vi "mainCryo With New Driver V1 and Cri Modified by Patiwet.vi"() -> ()   [LabVIEW 2012]
uses:
  SubVI/ProSCI Global.vi
  HTB/priorlibfilterout.vi
  <vilib>/Utility/config.llb/Write Key (I32).vi
  <vilib>/Utility/config.llb/Write Key (U32).vi
  <vilib>/Instr/_visa.llb/VISA Configure Serial Port (Instr).vi
  SubVI/ProSCI ConfigGlobal.vi
  <vilib>/Utility/config.llb/Read Key (U32).vi
  <vilib>/Utility/config.llb/Read Key (I32).vi
  <vilib>/Utility/config.llb/Read Key (Double).vi
  <vilib>/Utility/config.llb/Write Key (String).vi
  <vilib>/Utility/config.llb/Read Key (String).vi
  HTB/priorlibscanout.vi
  SubVI/ProSCI DebugGlobal.vi
  <vilib>/Utility/config.llb/NI_LVConfig.lvlib
panel:
  in  "stop":bool
  in  "port 2":i32=3
  in  "Case Constant\n(See Context Help) 3":bool
  in  "Case Constant\n(See Context Help) 2":bool
  in  "Case Constant\n(See Context Help)":bool=TRUE
  out "ExpTime":string
  out "ExpDate":string
  out "Event":i32(listbox)
  out "BotEdgePos":i32
  out "TopEdgePos":i32
  out "RtEdgePos":i32
  out "LtEdgePos":i32
  out "EdgeMarker":u8
  out "RobotIndexed":bool
  out "TotROI":i32
  out "TempXYArray":i32[](array[numeric])
  out "TileXYCoordinates":i32[][](array[numeric])
  out "Mag":u8
  out "Obj":u8
  out "CameraCounter":u32
  out "Br VISA Ref":refnum<visa-resource-name>="COM2"
  out "InGoHomeState":u32
  out "GoingHome":bool=TRUE
  out "CutCompXition":bool
  out "BaseDir":string
  in  "Tab Control":T1(tab)=enum."Imaging"
  in  "SampleThk":u32 max=70 step=1
  out "SecNumInFile":u32
  out "NotifyAbout":T2(ring)
  in  "Notify":bool
  out "UpdateMetadata":bool
  in  "PI":string
  in  "User":string
  out "ImageNow":bool
  out "TotalSessionCuts":u32
  out "SaveMetadata":bool
  in  "OpNotes":string
  in  "OpSliceThk":u16 max=50 step=1
  in  "OpSpecimen":string
  out "Present Cuts":u32
  in  "Total Cuts":u32
  out "Sequence Cut":bool
  in  "Image":bool
  out "IO Cut Comp":bool
  in  "FluoExpArray":dbl[](array[numeric])
  out "CutsCompletedLast":u32
  in  "ImageType":u16(ring) items=["Brightfield Only", "Fluorescence Only", "Brightfield & Fluorescence"]
  in  "ImageInterval":i32 min=0 max=25
  in  "IntervalMode":u16(ring) items=["Brightfield", "Fluorescence"]
  out "FlExpMem":dbl format="%#.3f"
  out "BrExpMem":dbl format="%#.3f"
  in  "FileNumStart":i32=1 min=0 max=10000
  in  "ImageSkipNum":i32 min=0 max=50
  in  "Capture Single Image":bool
  in  "ImageRepeatNum":u32=1 min=1
  out "FullFileName":string
  in  "SetFile Button":bool
  in  "FileNumbering":enum32{"Continuous", "With Section No."}(radio)=enum."With Section No."
  out "AutoXOffset":i32
  out "OffsetSlice":u32
  in  "OffsetPx":u32=1 min=1 step=1
  in  "Auto Offset":bool
  out "Pixel Size":dbl
  out "OffsetPresent":bool
  in  "ClearGlobalOffset":bool
  in  "StoreGlobalOffset":bool
  in  "Image ROI":bool
  in  "RobotStop":bool
  in  "BotEdge":bool
  in  "RightEdge":bool
  in  "LeftEdge":bool
  in  "TopEdge":bool
  out "Robot State":T3(ring)
  in  "RobotJog":bool
  in  "Magnification":string(combo)
  in  "Objective":string(combo)
  in  "Tile ROI":bool
  in  "MoveTo ROI":bool
  in  "Delete ROI":bool
  in  "Rename ROI":bool
  in  "Add ROI":bool
  in  "ROIName":string
  in  "ROI List":i32(listbox)
  in  "RobotFocus":bool
  in  "RobotImage":bool
  in  "RobotPark":bool
  in  "RobotIndex":bool
  out "RobotOnline":bool
  in  "RobotDisConnect":bool
  in  "RobotConnect":bool
  out "FlConnection":bool
  in  "Lamp Delay":dbl=2.0 min=0.5 max=5.0 step=0.1 format="%#.1f"
  in  "Shutter On":bool
  in  "BrDisonnectButton":bool
  in  "BrConnectButton":bool
  in  "FlDisonnectButton":bool
  in  "FlConnectButton":bool
  in  "FlIntensityLevel":u8(ring) items=["0%"=1, "11%"=2, "22%"=3, "33%"=4, "44%"=5, "55%"=6, "66%"=7, "77%"=8, "88%"=9, "100%"=10]
  out "BrLampStatus":T4(ring)
  out "BrConnection":bool
  out "BrFWVer":string
  in  "Lamp On":bool
  in  "Intensity":u8=100 max=100 step=10
  in  "Robot VISA Ref":refnum<visa-resource-name>
  out "Debug":string
  in  "Image Delay (sec)":dbl=2.0 format="%#_1g"
  in  "RobotIdx":bool
  in  "EProfile":bool
  in  "MinOverlap":bool
  out "LubBase":i32
  out "KnifeBase":i32
  in  "SaveFocusData":bool
  in  "Overlap":u8=15 min=5 max=90 step=1
  out "Camera Prog. OK":bool
  in  "Sys Reset":bool
  in  "Time Out (sec)":dbl=80.0 format="%#_1f"
  out "IO Fwd Stroke":bool
  in  "ResetLub":bool
  in  "ResetKnife":bool
  out "KnifeTime":i32
  out "LubTime":i32
  out "LubSetTime":u32=120 format="%#_3f"
  out "KnifeSetTime":u32=165 format="%#_3f"
  out "Lubricate":bool
  out "Change Knife":bool
  out "MBT Function: ErrorOut":errorcluster {"code" format="%.0x"}
  in  "AbortSeq":bool
  out "StXition":bool
  out "Current State":T5(ring)
  out "Imaging Done":bool
  in  "Single":bool
  in  "Sequence":bool
  in  "PauseReset":bool
  in  "Home":bool
  out "InFwdState":u32
  out "InDelayState":u32
  in  "Go Home Output":bool
  in  "Stop Cut Output":bool
  in  "Start Cut Output":bool
  out "Go Home":bool
  out "Stop Cut":bool
  out "Start Cut":bool
  out "IO EStop?":bool
  out "IO Comp Mode?":bool
  # "Op Exp Time - Remove Later"
  # "Emergency Stop?"
  # "In Computer Mode?"
  # "EVENT LOG"
  # "CONTROL"
  # "SETUP"
  # "STATUS"
  # "Experiment Details"
  # "Section Thickness"
  # "microns"
  # "Sample Thickness"
  # "mm"
  # "Notes"
  # "Cut Complete Signal"
  # "Sequence Cut"
  # "Total Cuts in Sequence"
  # "Image File #"
  # "Total Cuts This Session"
  # "Specimen"
  # "Cuts Completed"
  # "Only Sectioning"
  # "Section and Image"
  # "Skip Imaging every"
  # "Section(s)"
  # "Start File Numbering at"
  # "Base Image File Name"
  # "Images Per Section"
  # "Memorized BF Exposure Time"
  # "Memorized FL Exposure Time"
  # "msec"
  # "msec"
  # "Additional Fluo Exposures\n(Green Channel Only)"
  # "Select Image Type"
  # "Take"
  # "Image at Interval of"
  # "File Numbering"
  # "Robot Control"
  # "Scope Settings"
  # "Magnification"
  # "Objective"
  # "um"
  # "ROI/Tile Settings"
  # "New ROI"
  # "Selected ROI"
  # "FOV Offset"
  # "Manual"
  # "@"
  # "pixels"
  # "sections"
  # "Brightfield"
  # "Connection"
  # "Firmware Version"
  # "Lamp Unit Status"
  # "sec"
  # "Fluorescence"
  # "Connection"
  # "Firmware Version"
  # "Lamp Hours"
  # "Intensity Level"
  # "Mechanical"
  # "Miscellany"
  # "Change Knife every"
  # "IP: 169.254.0.101"
  # "Modbus TCP/IP"
  # "sections"
  # "Total Knife Run"
  # "sections"
  # "Change Knife?"
  # "Lubricate Machine every"
  # "sections"
  # "Total Lub Run Time"
  # "sec"
  # "Wait"
  # "sections"
  # "before Imaging"
  # "Lub Machine?"
  # "Tiling/ROI/Robot"
  # "Cut Complete Timeout"
  # "New Focus Data"
  # "seconds"
  # "Min Tile Overlap"
  # "%"
  # "Keep Overlap at Minimum"
  # "Robot Profile"
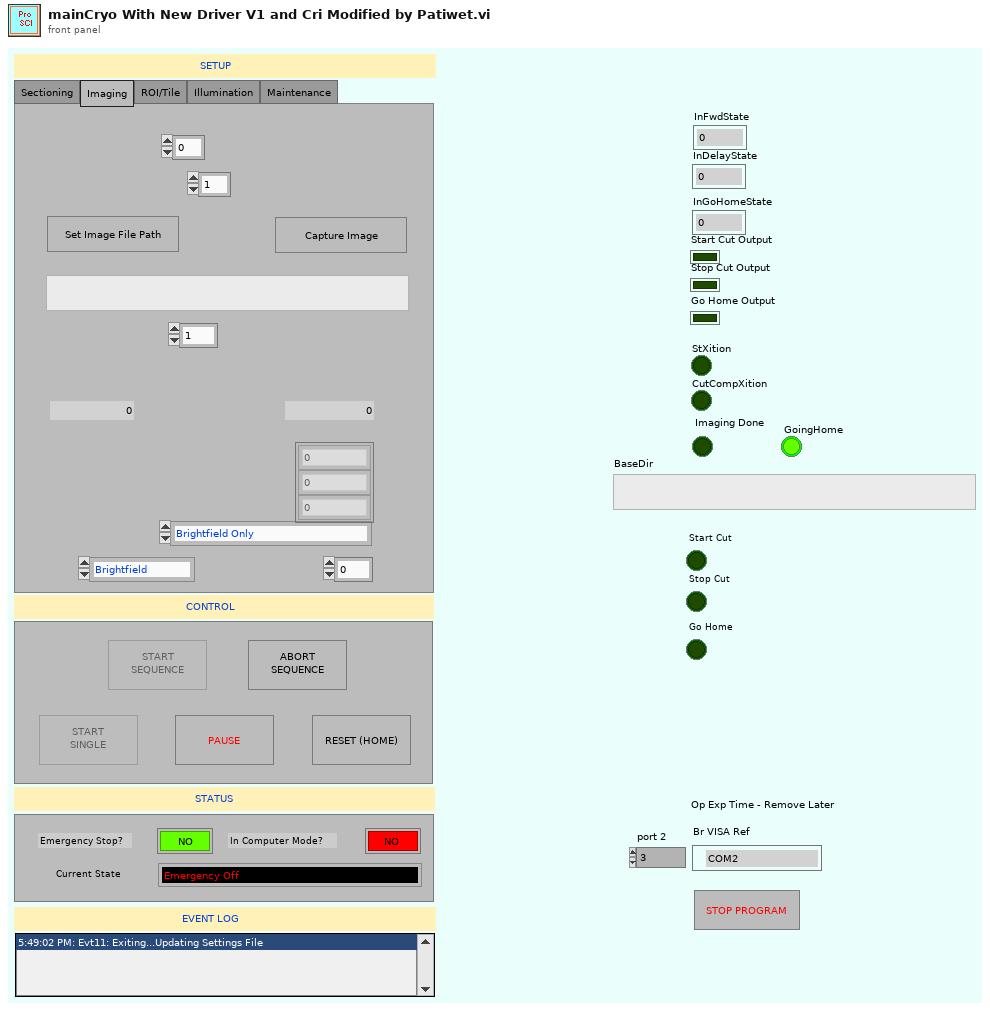
[diagram p1: front panel]
types:
  T1 = enum32{"Sectioning", "Imaging", "ROI/Tile", "Illumination", "Maintenance"}
  T2 = enum16{"Nothing", "In Progress", "Aborted", "Completed", "Sec TO"}
  T3 = enum16{"Idle", "Jog", "Indexing", "Parking", "Moving to Image", "Focusing", "Moving to ROI", "Not Indexed", "Offline"}
  T4 = enum16{"Undefined", "Connection Lost", "Not in Remote Mode", "Replace Bulb", "Lamp Unit OK"}
  T5 = enum16{"Emergency Off", "Manual", "Idle", "Spare 1", "Forward", "Pause", "Go Home", "Spare 2", "Cut Complete", "Imaging", "Spare 3", "Calculate Cuts", "Spare 4", "Time Out", "Delay Before Imaging"}
  T6 = enum16{"open", "open or create", "create or replace", "create", "open (read only)"}
  T7 = typedef "LVRectTypeDef.ctl" = cluster{"Left":i16, "Top":i16, "Right":i16, "Bottom":i16}
  T8 = typedef "NI_LVConfig.lvlib/Config Data RefNum.ctl" = refnum<k1>
  T9 = enum32{"existing file", "new file", "new or existing file", "existing dir", "new dir", "new or existing dir", "existing file (use LLBs)", "new file (use LLBs)", "new or existing file (use LLBs)", "new or existing file or directory (use LLBs)"}
  T10 = cluster{"PI":string, "User":string, "OpSpecimen":string, "OpSliceThk":u16, "OpNotes":string, "Image":bool}
  T11 = cluster{"ImageSkipNum":i32, "FileNumStart":i32, "FileNumbering":enum32{"Continuous", "With Section No."}, "FullFileName":string, "BaseDir":string, "ImageRepeatNum":u32, "BrExpMem":dbl, "FlExpMem":dbl, "ImageType":u16, "IntervalMode":u16, "ImageInterval":i32}
  T12 = cluster{"Obj":u8, "Mag":u8, "ItemNames":string[][], "TileXYCoordinates":i32[][], "TotROI":i32}
  T13 = cluster{"Time Out (sec)":dbl, "Overlap":u8, "MinOverlap":bool, "EProfile":bool, "Image Delay (sec)":dbl}
  T14 = enum16{"Undefined", "Focus", "XMin", "YMax", "XY", "Exposure"}
  T15 = enum16{"Idle", "Jog", "Indexing", "Parking", "Moving to Image", "Focusing", "Moving to ROI"}
  T16 = enum16{"Idle", "Jog", "Indexing", "Parking", "Moving to Image", "Focusing", "Moving to ROI", "Not Indexed"}
  T17 = enum16{"Add", "Delete", "Rename", "Update Tiles"}
  T18 = enum16{"Undefined", "Focus", "XMin", "YMax", "XY"}
  T19 = enum16{"Nothing", "In Progress", "Aborted", "Completed"}
  T20 = cluster{"TileCoordinates":i32[][], "XTiles":u16, "YTiles":u16, "TileSuffix":string[], "XOverlap":dbl, "YOverlap":dbl}
  T21 = cluster{"User":string, "PI":string, "OpSpecimen":string, "OpSliceThk":u16, "OpNotes":string, string, string}
  T22 = enum32{"invalid app kind", "Development System", "Run Time System", "Student Edition", "Embedded LabVIEW", "Evaluation", "Custom"}
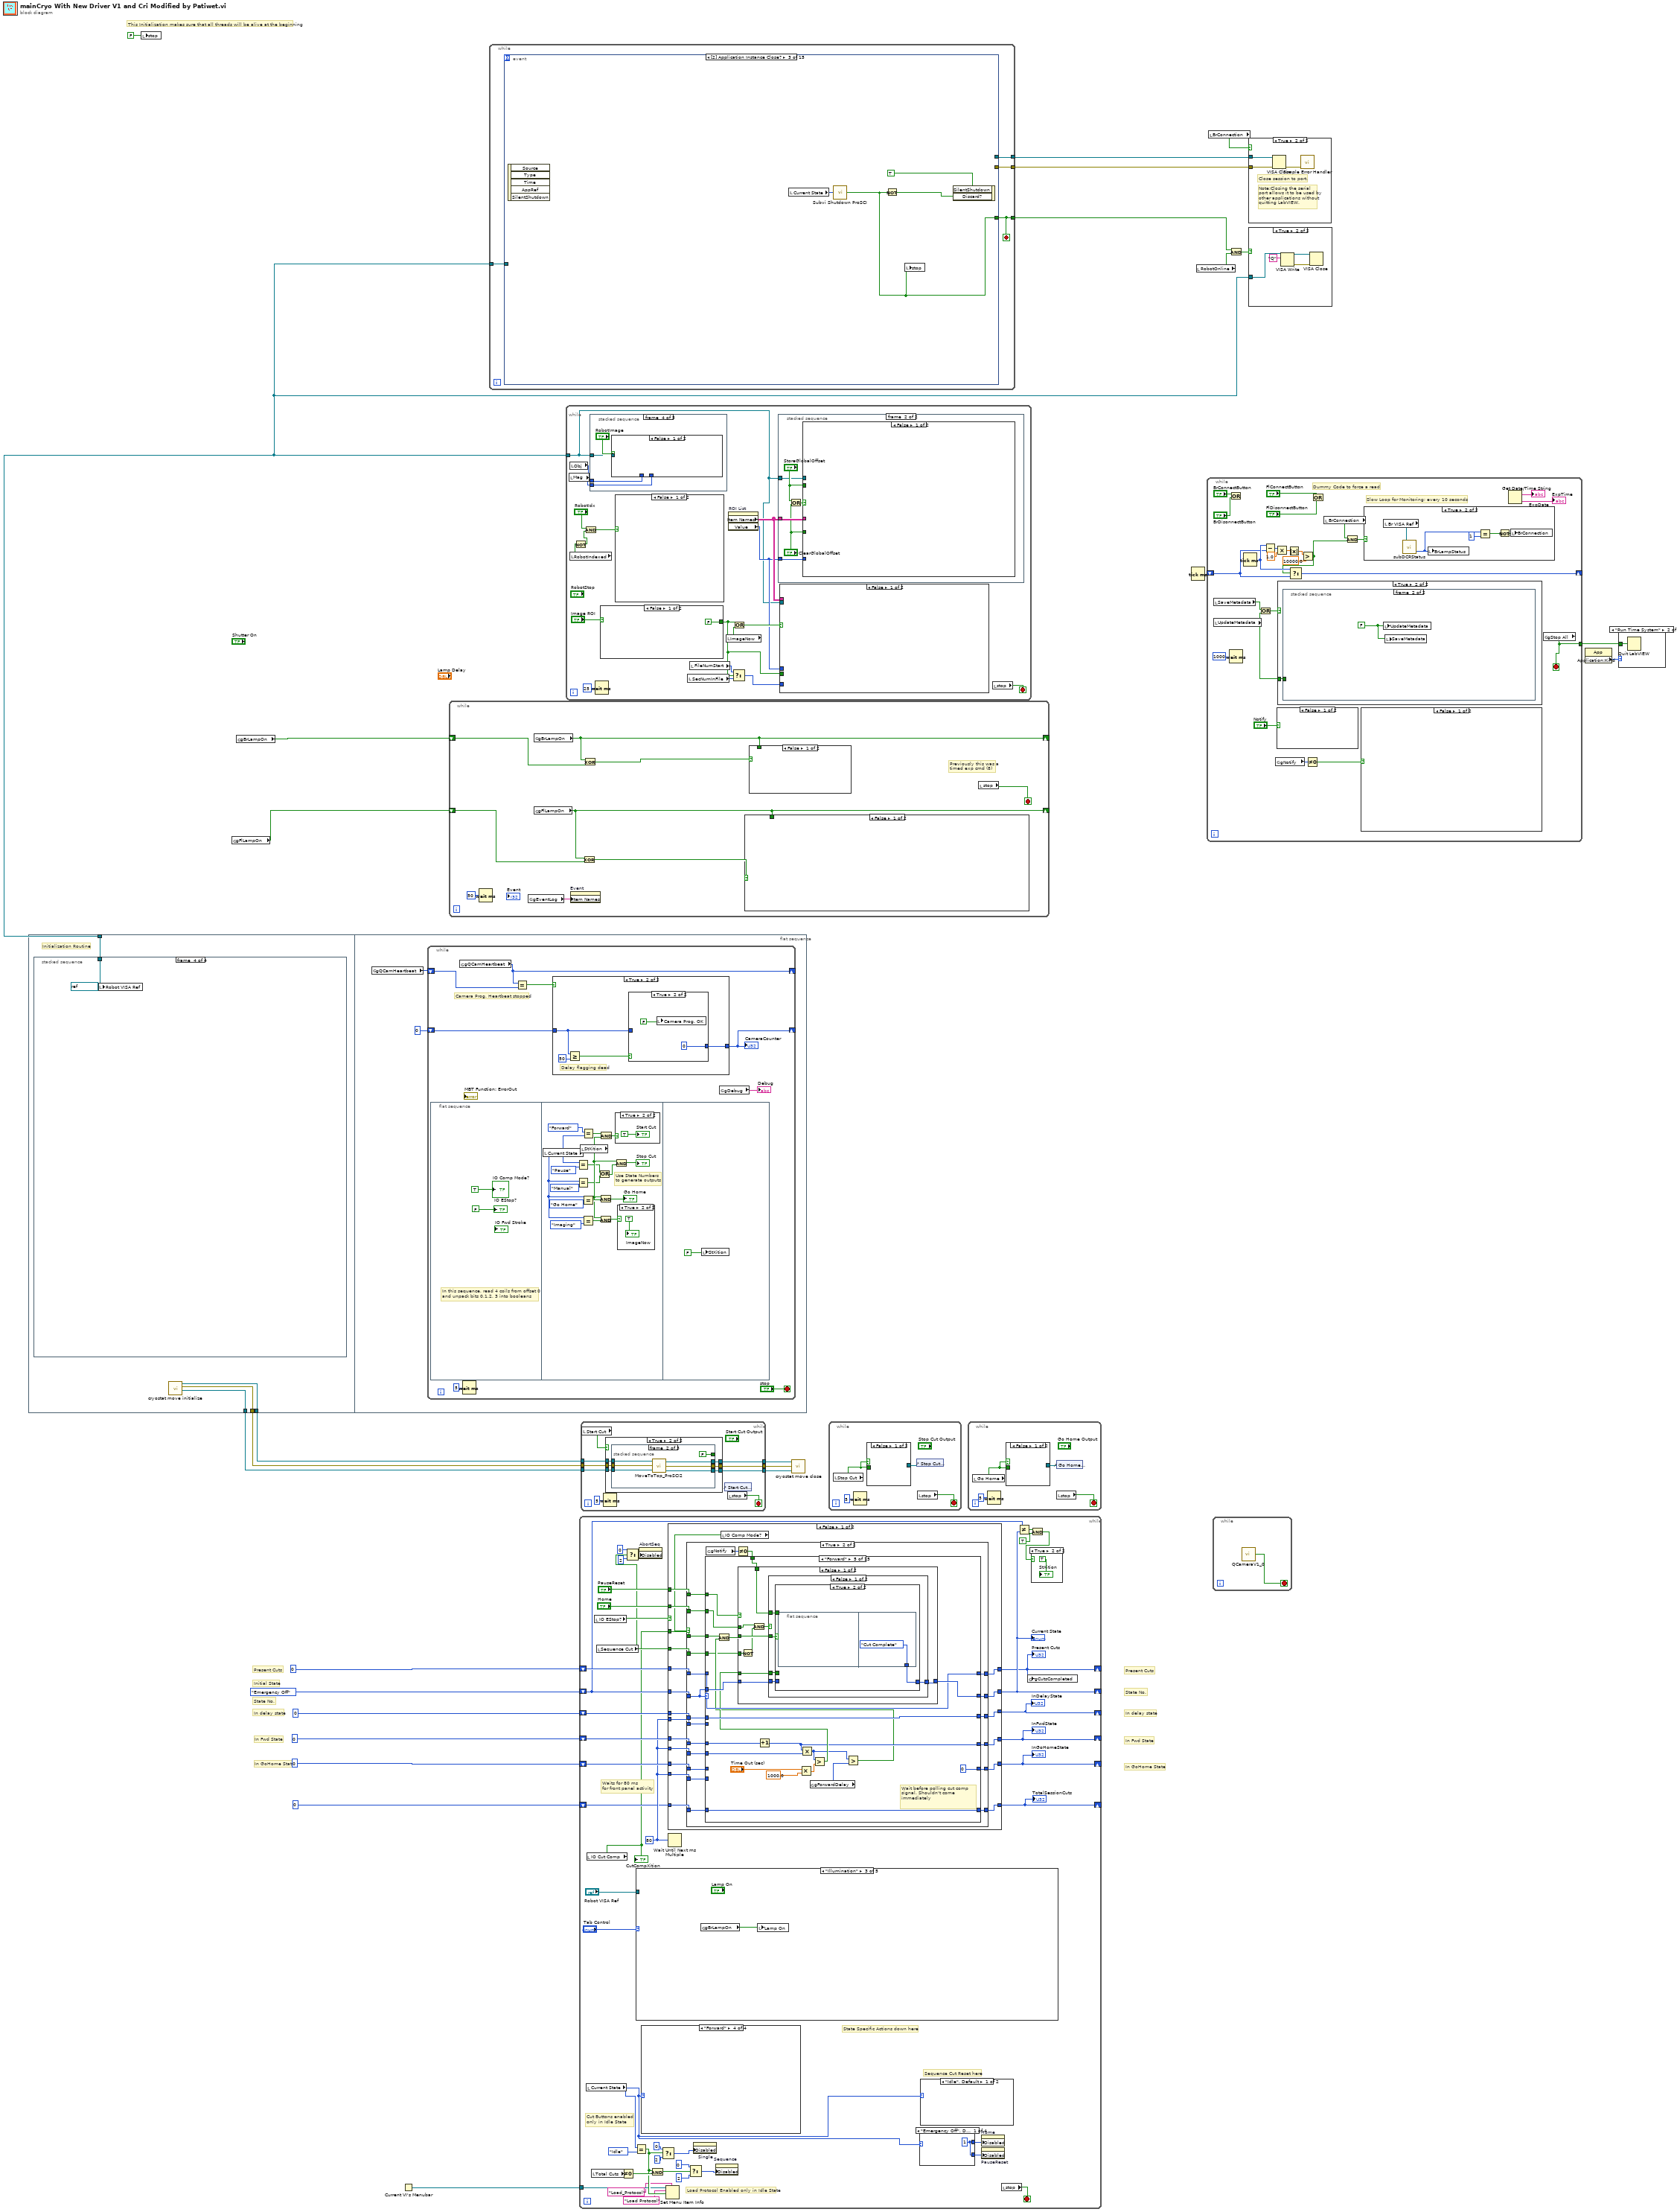
[diagram p0: block diagram]
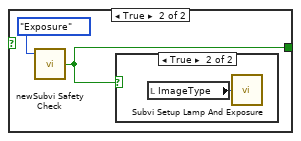
[diagram p5: hidden frame]
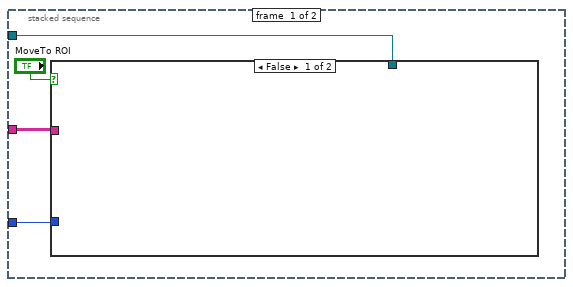
[diagram p7: hidden frame]
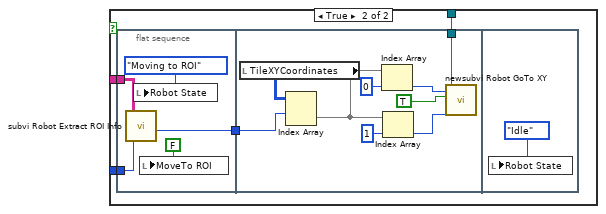
[diagram p8: hidden frame]
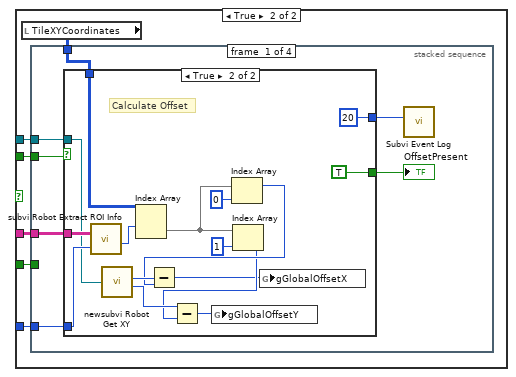
[diagram p9: hidden frame]
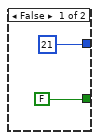
[diagram p10: hidden frame]
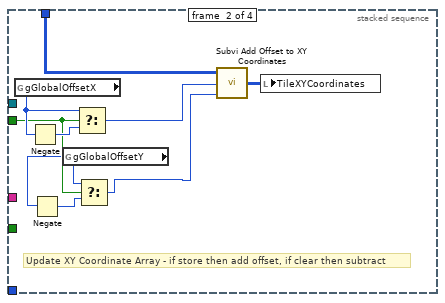
[diagram p11: hidden frame]
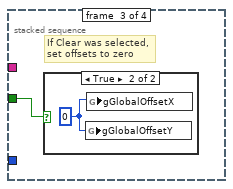
[diagram p12: hidden frame]
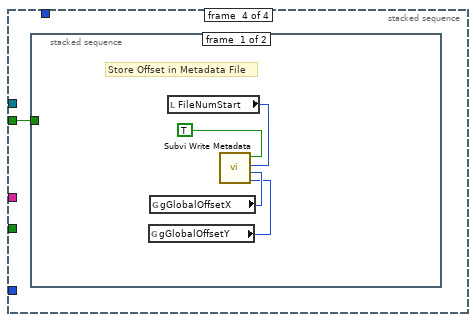
[diagram p14: hidden frame]
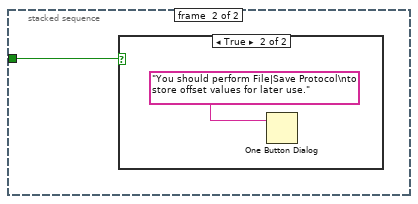
[diagram p15: hidden frame]
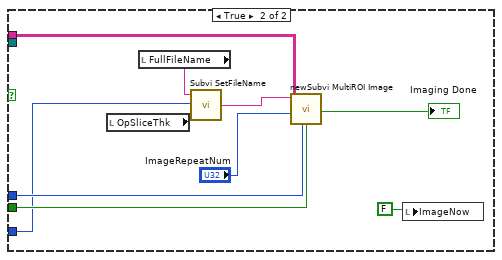
[diagram p17: hidden frame]
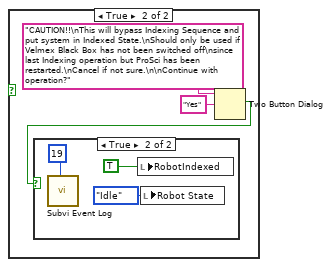
[diagram p18: hidden frame]
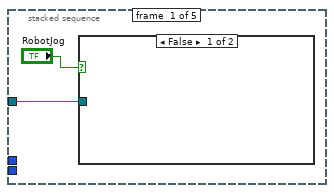
[diagram p20: hidden frame]
diagram:
  # "This Initialization makes sure that all threads will be alive at the beginning"
  # "In GoHome State"
  # "In GoHome State"
  # "In Fwd State"
  # "In Fwd State"
  # "Present Cuts"
  # "Present Cuts"
  # "State No."
  # "In delay state"
  # "In delay state"
  # "State No."
  # "Initial State"
  n1 = flat-sequence {
    tunnel: [w30] -> w9
    tunnel: [w29] -> w6
    tunnel: [w28] -> w5
    tunnel: [w27] -> w4
    frame #0 {
      # "Initialization Routine"
      n2 = stacked-sequence {
        tunnel: [_ _ _ w107] -> w30
        frame #0 {
          w43 = i16 0
          # "Open Logfile"
          # "Window Size, Title"
          n3 = property class="VI"() -> ("Front Panel Window:Window Bounds"=w39:T7)  [unwired: 2 in, 2 out]
          n4 = Current VI's Path() -> (path=w34:path)
          n5 = Strip Path(path=w34) -> (stripped path=w32:path)  [unwired: 1 out]
          n6 = Strip Path(path=w32) -> (stripped path=w31:path)  [unwired: 1 out]
          n7 = Unbundle(w39) -> ("Right"=w42:i16, "Bottom"=w41:i16)  [unwired: 2 out]
          n8 = Bundle(w43, w43, "Right"=w42, "Bottom"=w41) -> (w40:cluster{i16, i16, "Right":i16, "Bottom":i16})  [unwired: 1 out]
          n9 = Concatenate Strings("Pro-SCI" ("string"), " - Untitled" ("string")) -> (w46:string)
          n10 = property class="VI"("Front Panel Window:Window Bounds"=w40, "Front Panel Window:Title"=w46) -> ()  [unwired: 2 in, 2 out]
          n11 = call "Subvi SetLogFileName.vi"("LogFileMax"=u8 10 ("y"), "BaseAppPath"=w31, "LogFileBaseName"="ProSCILog") -> ("LogFilePath"=w33:path)
          n12 = call <vilib>:"Open_Create_Replace File.vi"("function (open:0)"=T6."open or create", "file path"=w33) -> ("refnum"=w37:refnum<file>)  [unwired: 4 in, 5 out]
          n13 = global write "ProSCI Global.vi" "gLogFileRef"(w37) -> ()
        }
        frame #1 {
          w50 = "D:\\Default" ("string")
          w55 = string[] [] ("Item Names")
          w48 = u8 0 ("gAppsStopped")
          w60 = FALSE
          w62 = u8 0 ("Disabled")
          n14 = local write "TileXYCoordinates"(i32[][] [] ("TileXYCoordinates")) -> ()
          n15 = local write "TempXYArray"(i32[] [] ("TempXYArray")) -> ()
          n16 = global write "ProSCI Global.vi" "gStop All"(w60) -> ()
          n17 = global write "ProSCI Global.vi" "gCutSequenceOn"(w60) -> ()
          n18 = local write "BaseDir"(w50) -> ()
          n19 = property on="ROI List" class="MCListbox (strict)"("Item Names"=string[][] []) -> ()  [unwired: 2 in, 2 out]
          n20 = global write "ProSCI Global.vi" "gBaseDir"(w50) -> ()
          n21 = Concatenate Strings(w50, "\\CryoDefault" ("string")) -> (w51:string)
          n22 = local write "Tab Control"(T1."Sectioning" ("Tab Control")) -> ()
          n23 = local write "FullFileName"(w51) -> ()
          n24 = global write "ProSCI Global.vi" "gBaseFile"(w51) -> ()
          n25 = property on="TopEdge" class="Bool"("Visible"=w60) -> ()  [unwired: 2 in, 2 out]
          n26 = property on="BotEdge" class="Bool"("Visible"=w60) -> ()  [unwired: 2 in, 2 out]
          n27 = property on="Magnification" class="CmbBox"("Value"="0" ("Magnification")) -> ()  [unwired: 2 in, 2 out]
          n28 = global write "ProSCI Global.vi" "gEventLog"(w55) -> ()
          n29 = property on="Event" class="LstBox (strict)"("Item Names"=w55) -> ()  [unwired: 2 in, 2 out]
          n30 = property on="RightEdge" class="Bool"("Visible"=w60) -> ()  [unwired: 2 in, 2 out]
          n31 = property on="LeftEdge" class="Bool"("Visible"=w60) -> ()  [unwired: 2 in, 2 out]
          n32 = property on="Objective" class="CmbBox"("Value"="0" ("Objective")) -> ()  [unwired: 2 in, 2 out]
          n33 = To Double Precision Float(number=w48) -> (double precision float=w49:dbl)
          n34 = local write "FlIntensityLevel"(10) -> ()
          n35 = property on="FlConnectButton" class="Bool (strict)"("Disabled"=w62) -> ()  [unwired: 2 in, 2 out]
          n36 = property on="BrDisonnectButton" class="Bool (strict)"("Disabled"=w62) -> ()  [unwired: 2 in, 2 out]
          n37 = property on="BrConnectButton" class="Bool (strict)"("Disabled"=w62) -> ()  [unwired: 2 in, 2 out]
          n38 = property on="FlDisonnectButton" class="Bool (strict)"("Disabled"=w62) -> ()  [unwired: 2 in, 2 out]
          n39 = global write "ProSCI Global.vi" "gExpTimeSendToCamera"(w49) -> ()
          n40 = local write "EdgeMarker"(w48) -> ()
          n41 = global write "ProSCI Global.vi" "gAppsStopped"(w48) -> ()
          n42 = local write "TotROI"(w48) -> ()
          "Robot State" <- T3."Offline" ("Robot State")
        }
        frame #2 {
          w75 = "Robot" ("section")
          w87 = "Mechanical" ("section")
          # "This number should always be negative"
          # "Row = Magnification\nCol = Objective"
          # "in microns"
          # "90x"
          # "7x"
          # "1.0X"
          # "0.3X"
          # "Later replace this part by reading the same settings from Settings file"
          # "Read from Settings File"
          n43 = String To Path(string="C:\\Program Files\\ProSCI\\ProSciSettings.ini") -> (path=w102:path)
          n44 = call <vilib>:"Open Config Data (compatibility).vi"("create file if necessary (T)"=FALSE ("create file if necessary? (T)"), "configuration file path"=w102) -> ("error out"=w98:errorcluster, "refnum"=w100:T8)  [unwired: 7 in, 1 out]
          n45 = call-poly <vilib>:"Read Key.vi"("section"=w87, "error in (no error)"=w98, "default value"=u32 0, "key"="ChangeKnife", "refnum"=w100) -> ("error out"=w91:errorcluster, "value"=→"KnifeSetTime":u32, "refnum out"=w92:T8)  [unwired: 4 out]
          n46 = call-poly <vilib>:"Read Key.vi"("section"=w87, "error in (no error)"=w91, "default value"=0, "key"="KnifeRun", "refnum"=w92) -> ("error out"=w89:errorcluster, "value"=w79:i32, "refnum out"=w90:T8)  [unwired: 4 out]
          "KnifeBase" <- w79
          n47 = global write "ProSCI ConfigGlobal.vi" "gCfgPixelSize"(dbl[][] [[52.0, 15.6], [41.2, 11.0], [29.3, 8.8], [24.0, 7.2], [18.0, 5.4], [15.4, 4.6], [11.7, 3.5], [9.6, 2.9], [7.1, 2.1], [5.3, 1.6], [4.0, 1.2]] ("array")) -> ()
          n48 = local write "KnifeTime"(w79) -> ()
          n49 = call-poly <vilib>:"Read Key.vi"("section"=w87, "error in (no error)"=w89, "default value"=u32 0, "key"="LubMachine", "refnum"=w90) -> ("error out"=w83:errorcluster, "value"=→"LubSetTime":u32, "refnum out"=w86:T8)  [unwired: 4 out]
          n50 = call-poly <vilib>:"Read Key.vi"("section"=w87, "error in (no error)"=w83, "default value"=0, "key"="LubRun", "refnum"=w86) -> ("error out"=w76:errorcluster, "value"=w80:i32, "refnum out"=w77:T8)  [unwired: 4 out]
          "LubBase" <- w80
          n51 = call-poly <vilib>:"Read Key.vi"("section"=w75, "error in (no error)"=w76, "default value"=6.35, "key"="MicronPerStep" ("section"), "refnum"=w77) -> ("error out"=w73:errorcluster, "value"=w70:dbl, "refnum out"=w74:T8)  [unwired: 4 out]
          n52 = global write "ProSCI ConfigGlobal.vi" "gCfgMicronPerStep"(w70) -> ()
          n53 = call-poly <vilib>:"Read Key.vi"("section"=w75, "error in (no error)"=w73, "default value"=-0.267949, "key"="MicronPerMicronThickness" ("section"), "refnum"=w74) -> ("error out"=w66:errorcluster, "value"=w64:dbl, "refnum out"=w67:T8)  [unwired: 4 out]
          n54 = Greater Or Equal To 0?(x=w64) -> (x >= 0?=w65:bool)
          n55 = call <vilib>:"Close Config Data.vi"("error in (no error)"=w66, "write file if changed (T)"=FALSE ("write configuration file? (T)"), "refnum"=w67) -> ()  [unwired: 9 out]
          n56 = case shown="True" w65 {
            tunnel: w64 -> [w104 w106]
            tunnel: [w104 w105] -> w63
            frame False {
            }
            frame True {
              n57 = Negate(x=w106) -> (-x=w105:dbl)
            }
          }
          n58 = global write "ProSCI ConfigGlobal.vi" "gCfgMicronPerMicronThickness"(w63) -> ()
          n59 = local write "LubTime"(w80) -> ()
        }
        frame #3 {
          w107 = refnum<visa-resource-name> "COM8" ("Robot VISA Ref")
          n60 = local write "Robot VISA Ref"(w107) -> ()
        }
      }
      n61 = call "cryostat move initialize.vi"() -> ("VISA resource name out"=w27:refnum<visa-resource-name>, "error out 2"=w28:errorcluster, "task out"=w29:refnum<k21>)  [unwired: 8 in, 1 out]
    }
    frame #1 {
      n62 = global read "ProSCI Global.vi" "gQCamHeartbeat"() -> (w109:u32)
      n63 = while {
        shift-right: [w111] -> _
        shift-left: w109 -> [w115]
        shift-right: [w114] -> _
        shift-left: 0 -> [w113]
        stop <- "stop" stop-if-true
        # "Camera Prog. Heartbeat stopped"
        n64 = flat-sequence {
          frame #0 {
            # "In this sequence, read 4 coils from offset 0\nand unpack bits 0,1,2, 3 into booleans"
            "IO Comp Mode?" <- TRUE ("UseTCP")
            "IO EStop?" <- FALSE ("UseTCP")
          }
          frame #1 {
            # "Use State Numbers\nto generate outputs"
            n65 = local read "Current State"() -> (w135:T5)
            n66 = Equal?(x=w135, y=T5."Pause") -> (x = y?=w133:bool)
            n67 = Equal?(x=w135, y=T5."Manual") -> (x = y?=w132:bool)
            n68 = local read "StXition"() -> (w137:bool)
            n69 = Equal?(x=w135, y=T5."Go Home") -> (x = y?=w142:bool)
            n70 = Equal?(x=w135, y=T5."Imaging") -> (x = y?=w138:bool)
            n71 = Equal?(x=T5."Forward", y=w135) -> (x = y?=w145:bool)
            n72 = Or(x=w133, y=w132) -> (x .or. y?=w134:bool)
            n73 = And(x=w137, y=w142) -> (x .and. y?=→"Go Home":bool)
            n74 = And(x=w137, y=w138) -> (x .and. y?=w131:bool)
            n75 = And(x=w145, y=w137) -> (x .and. y?=w130:bool)
            n76 = And(x=w137, y=w134) -> (x .and. y?=→"Stop Cut":bool)
            n77 = case shown="True" w130 {
              frame False {
              }
              frame True {
                "Start Cut" <- TRUE
              }
            }
            n78 = case shown="True" w131 {
              frame False {
              }
              frame True {
                "ImageNow" <- TRUE
              }
            }
          }
          frame #2 {
            n79 = local write "StXition"(FALSE) -> ()
          }
        }
        n80 = global read "ProSCI Global.vi" "gQCamHeartbeat"() -> (w111:u32)
        n81 = Wait (ms)(milliseconds to wait=u32 5) -> ()  [unwired: 1 out]
        n82 = Equal?(x=w111, y=w115) -> (x = y?=w112:bool)
        n83 = case shown="True" w112 {
          tunnel: [0 w121] -> w114
          tunnel: w113 -> [_ w120]
          frame False {
            "Camera Prog. OK" <- TRUE
          }
          frame True {
            # "Delay flagging dead"
            n84 = Greater Or Equal?(x=w120, y=u32 50) -> (x >= y?=w122:bool)
            n85 = case shown="True" w122 {
              tunnel: [w124 0] -> w121
              tunnel: w120 -> [w125 _]
              frame False {
                n86 = Increment(x=w125) -> (x+1=w124:i32)
              }
              frame True {
                n87 = local write "Camera Prog. OK"(FALSE) -> ()
              }
            }
          }
        }
        "CameraCounter" <- w114
        n88 = global read "ProSCI DebugGlobal.vi" "gDebug"() -> (→"Debug":string)
      }
    }
  }
  n89 = local write "stop"(FALSE) -> ()
  n90 = global read "ProSCI Global.vi" "gFlLampOn"() -> (w7:bool)
  n91 = global read "ProSCI Global.vi" "gBrLampOn"() -> (w19:bool)
  n92 = Current VI's Menubar() -> (w16:refnum<k9>)
  n93 = while {
    shift-right: [w156] -> _
    shift-left: w19 -> [w155]
    shift-right: [w150] -> _
    shift-left: w7 -> [w152]
    stop <- w153 stop-if-true
    # "Previously this was a\ntimed exp cmd (8)"
    n94 = Wait (ms)(milliseconds to wait=u32 50) -> ()  [unwired: 1 out]
    n95 = global read "ProSCI Global.vi" "gEventLog"() -> (w154:string[])
    n96 = global read "ProSCI Global.vi" "gBrLampOn"() -> (w156:bool)
    n97 = global read "ProSCI Global.vi" "gFlLampOn"() -> (w150:bool)
    n98 = property on="Event" class="LstBox (strict)"("Item Names"=w154) -> ()  [unwired: 2 in, 2 out]
    n99 = Exclusive Or(1:w152, 2:w150) -> (0:w151:bool)
    n100 = Exclusive Or(1:w155, 2:w156) -> (0:w157:bool)
    n101 = case shown="False" w151 {
      tunnel: w150 -> [_ w159]
      frame False {
      }
      frame True {
        n102 = case shown="True" w159 {
          tunnel: w159 -> [_ w164]
          frame False {
            n103 = flat-sequence {
              frame #0 {
                # "Close Shutter"
                n104 = global read "priorlibfilterout.vi" "PRIORLib.IFilterOut"() -> (w161:refnum<k7>)
                n105 = call "IFilterMoveToPosition.vi"("Wheel"=1, "filter"=u8 1 ("f"), "PRIORLib.IFilterIn"=w161) -> ()  [unwired: 3 out]
              }
            }
          }
          frame True {
            n106 = flat-sequence {
              tunnel: w164 -> [_]
              tunnel: [w166] -> w163
              tunnel: w163 -> [w170]
              frame #0 {
                # "Open Shutter with Chosen Intensity"
                n107 = global read "priorlibfilterout.vi" "PRIORLib.IFilterOut"() -> (w166:refnum<k7>)
                n108 = call "IFilterMoveToPosition.vi"("Wheel"=1, "filter"="FlIntensityLevel", "PRIORLib.IFilterIn"=w166) -> ()  [unwired: 3 out]
              }
              frame #1 {
                # "Set Excitation\nFilters"
                n109 = global read "ProSCI Global.vi" "gFLExcitationFilter"() -> (w169:i8)
                n110 = call "IFilterMoveToPosition.vi"("Wheel"=2, "filter"=w169, "PRIORLib.IFilterIn"=w170) -> ()  [unwired: 3 out]
              }
            }
          }
        }
      }
    }
    n111 = case shown="False" w157 {
      tunnel: w156 -> [_ w172]
      frame False {
      }
      frame True {
        n112 = local read "Br VISA Ref"() -> (w171:refnum<visa-resource-name>)
        n113 = call "subVI DCR3 Lamp OnOff.vi"("Lamp"=w172, "VISA resource name"=w171) -> ()  [unwired: 1 out]
      }
    }
    n114 = local read "stop"() -> (w153:bool)
  }
  n115 = while {
    tunnel: [w175] -> w21
    tunnel: [w176] -> w20
    tunnel: w9 -> [w174]
    tunnel: [w173] -> w12
    stop <- w173 stop-if-true
    n116 = event shown="[2] Application Instance Close?" {
      selector: _ -> [_ _ _ _ _ _ _ _ _ _ _ _ _ _ _]
      dyn-events: _ -> [_ _ _ _ _ _ _ _ _ _ _ _ _ _ _]
      timeout: _ -> [_ _ _ _ _ _ _ _ _ _ _ _ _ _ _]
      tunnel: [_ _ w381 _ _ _ _ _ _ w426 _ _ _ _ _] -> w173
      tunnel: [_ _ _ _ _ _ _ _ _ _ w431 _ _ _ _] -> w175
      tunnel: [_ _ _ _ _ _ _ _ _ _ w430 _ _ _ _] -> w176
      tunnel: w174 -> [_ _ _ _ _ _ _ _ _ _ _ w446 _ _ _]
      event Menu Selection (User) {
        n117 = event-data() -> ("ItemTag"=w177:string)  [unwired: 6 out]
        n118 = case shown="\"Load_Protocol\", \"Save_Protocol\"" w177 {
          tunnel: w177 -> [_ w180 _ _]
          frame Default {
            n119 = One Button Dialog(message="Coming Soon!") -> ()  [unwired: 2 out]
          }
          frame "Load_Protocol", "Save_Protocol" {
            n120 = local read "RobotIndexed"() -> (w179:bool)
            n121 = case shown="True" w179 {
              tunnel: w180 -> [_ w205]
              frame False {
                n122 = call "Subvi Event Log.vi"("EventNum"=u32 12) -> ()  [unwired: 1 in]
              }
              frame True {
                w198 = "ProSCI Protocol" ("y")
                w206 = "Enter Filename:"  # Prompt
                n123 = stacked-sequence {
                  tunnel: ["Sectioning" ("key") _ _ _ _] -> w197
                  tunnel: [w210 _ _ _ _] -> w196
                  tunnel: [_ "Imaging" ("key") _ _ _] -> w195
                  tunnel: [_ w218 _ _ _] -> w194
                  tunnel: [_ _ "ROI" ("key") _ _] -> w193
                  tunnel: [_ _ w232 _ _] -> w192
                  tunnel: [_ _ _ "Illumination" ("key") _] -> w191
                  tunnel: [_ _ _ w240 _] -> w190
                  tunnel: [_ _ _ _ "Maintenance" ("key")] -> w189
                  tunnel: [_ _ _ _ w245] -> w188
                  tunnel: [_ _ _ _ w244] -> w186
                  tunnel: [_ _ _ w239 _] -> w185
                  tunnel: [_ _ w231 _ _] -> w184
                  tunnel: [_ w217 _ _ _] -> w183
                  tunnel: [w209 _ _ _ _] -> w182
                  frame #0 {
                    # "Sectioning Tab"
                    n124 = local read "OpSpecimen"() -> (w215:string)
                    n125 = local read "OpSliceThk"() -> (w214:u16)
                    n126 = local read "OpNotes"() -> (w213:string)
                    n127 = local read "Image"() -> (w212:bool)
                    n128 = local read "User"() -> (w216:string)
                    n129 = local read "PI"() -> (w208:string)
                    n130 = Bundle("PI"=w208, "User"=w216, "OpSpecimen"=w215, "OpSliceThk"=w214, "OpNotes"=w213, "Image"=w212) -> (w209:T10)  [unwired: 1 out]
                    n131 = Flatten To String(anything=w209) -> (data string=w210:string)  [unwired: 1 in, 4 out]
                  }
                  frame #1 {
                    # "Imaging Tab"
                    n132 = local read "ImageSkipNum"() -> (w230:i32)
                    n133 = local read "FileNumbering"() -> (w228:enum32{"Continuous", "With Section No."})
                    n134 = local read "FullFileName"() -> (w227:string)
                    n135 = local read "ImageRepeatNum"() -> (w225:u32)
                    n136 = local read "FileNumStart"() -> (w229:i32)
                    n137 = local read "BrExpMem"() -> (w224:dbl)
                    n138 = local read "FlExpMem"() -> (w223:dbl)
                    n139 = local read "IntervalMode"() -> (w221:u16)
                    n140 = local read "ImageType"() -> (w222:u16)
                    n141 = local read "ImageInterval"() -> (w220:i32)
                    n142 = local read "BaseDir"() -> (w226:string)
                    n143 = Bundle("ImageSkipNum"=w230, "FileNumStart"=w229, "FileNumbering"=w228, "FullFileName"=w227, "BaseDir"=w226, "ImageRepeatNum"=w225, "BrExpMem"=w224, "FlExpMem"=w223, "ImageType"=w222, "IntervalMode"=w221, "ImageInterval"=w220) -> (w217:T11)  [unwired: 1 out]
                    n144 = Flatten To String(anything=w217) -> (data string=w218:string)  [unwired: 1 in, 4 out]
                  }
                  frame #2 {
                    # "ROI Tab"
                    n145 = local read "TileXYCoordinates"() -> (w235:i32[][])
                    n146 = local read "Obj"() -> (w238:u8)
                    n147 = local read "Mag"() -> (w237:u8)
                    n148 = local read "TotROI"() -> (w234:i32)
                    n149 = property on="ROI List" class="MCListbox (strict)"() -> ("Item Names"=w236:string[][])  [unwired: 2 in, 2 out]
                    n150 = Bundle("Obj"=w238, "Mag"=w237, "ItemNames"=w236, "TileXYCoordinates"=w235, "TotROI"=w234) -> (w231:T12)  [unwired: 1 out]
                    n151 = Flatten To String(anything=w231) -> (data string=w232:string)  [unwired: 1 in, 4 out]
                  }
                  frame #3 {
                    # "Illumination Tab"
                    n152 = local read "Lamp Delay"() -> (w242:dbl)
                    n153 = Bundle("Lamp Delay"=w242) -> (w239:cluster{"Lamp Delay":dbl})  [unwired: 1 in]
                    n154 = Flatten To String(anything=w239) -> (data string=w240:string)  [unwired: 1 in, 4 out]
                  }
                  frame #4 {
                    # "Maintenance Tab"
                    n155 = local read "Time Out (sec)"() -> (w250:dbl)
                    n156 = local read "MinOverlap"() -> (w248:bool)
                    n157 = local read "EProfile"() -> (w247:bool)
                    n158 = local read "Overlap"() -> (w249:u8)
                    n159 = local read "Image Delay (sec)"() -> (w243:dbl)
                    n160 = Bundle("Time Out (sec)"=w250, "Overlap"=w249, "MinOverlap"=w248, "EProfile"=w247, "Image Delay (sec)"=w243) -> (w244:T13)  [unwired: 1 out]
                    n161 = Flatten To String(anything=w244) -> (data string=w245:string)  [unwired: 1 in, 4 out]
                  }
                }
                n162 = Equal?(x=w205, y="Load_Protocol") -> (x = y?=w187:bool)
                n163 = Select(t=T9."existing file" ("select mode (2)"), s=w187, f=T9."new or existing file" ("select mode (2)")) -> (s? t:f=w201:T9)
                n164 = call <vilib>:"compatFileDialog.vi"("pattern label"=w198, "prompt"=w206, "pattern"="*.psc", "select mode (2)"=w201) -> ("cancelled"=w200:bool, "path"=w207:path)  [unwired: 3 in, 3 out]
                n165 = case shown="False" w200 {
                  tunnel: w207 -> [w255 _]
                  tunnel: w187 -> [w251 _]
                  tunnel: w198 -> [w271 _]
                  tunnel: w197 -> [w270 _]
                  tunnel: w196 -> [w269 _]
                  tunnel: w195 -> [w268 _]
                  tunnel: w194 -> [w267 _]
                  tunnel: w193 -> [w266 _]
                  tunnel: w192 -> [w265 _]
                  tunnel: w191 -> [w264 _]
                  tunnel: w190 -> [w263 _]
                  tunnel: w189 -> [w262 _]
                  tunnel: w188 -> [w261 _]
                  tunnel: w186 -> [w260 _]
                  tunnel: w185 -> [w259 _]
                  tunnel: w184 -> [w258 _]
                  tunnel: w183 -> [w257 _]
                  tunnel: w182 -> [w256 _]
                  frame False {
                    n166 = Not(x=w251) -> (.not. x?=w252:bool)
                    n167 = call <vilib>:"Open Config Data (compatibility).vi"("create file if necessary (T)"=w252, "configuration file path"=w255) -> ("error out"=w253:errorcluster, "refnum"=w272:T8)  [unwired: 7 in, 1 out]
                    n168 = Path To String(path=w255) -> (string=w254:string)
                    n169 = case shown="True" w251 {
                      tunnel: w272 -> [w276 w308]
                      tunnel: w271 -> [w290 w323]
                      tunnel: w270 -> [w298 w324]
                      tunnel: w269 -> [w297 _]
                      tunnel: w268 -> [w296 w321]
                      tunnel: w267 -> [w295 _]
                      tunnel: w266 -> [w294 w320]
                      tunnel: w265 -> [w293 _]
                      tunnel: w264 -> [w292 w319]
                      tunnel: w263 -> [w291 _]
                      tunnel: w262 -> [w289 w318]
                      tunnel: w261 -> [w288 _]
                      tunnel: w260 -> [_ w313]
                      tunnel: w259 -> [_ w312]
                      tunnel: w258 -> [_ w311]
                      tunnel: w257 -> [_ w310]
                      tunnel: w256 -> [_ w309]
                      tunnel: w254 -> [w286 w301]
                      tunnel: w253 -> [w277 w299]
                      frame False {
                        # "Save Protocol"
                        n170 = Concatenate Strings("Saving Protocol in " ("string"), w286) -> (w284:string)
                        n171 = call-poly <vilib>:"Write Key.vi"("section"=w290, "error in (no error)"=w277, "value"=w297, "key"=w298, "refnum"=w276) -> ("error out"=w281:errorcluster)  [unwired: 1 in, 5 out]
                        n172 = call-poly <vilib>:"Write Key.vi"("section"=w290, "error in (no error)"=w281, "value"=w295, "key"=w296, "refnum"=w276) -> ("error out"=w279:errorcluster)  [unwired: 1 in, 5 out]
                        n173 = call-poly <vilib>:"Write Key.vi"("section"=w290, "error in (no error)"=w279, "value"=w293, "key"=w294, "refnum"=w276) -> ("error out"=w280:errorcluster)  [unwired: 1 in, 5 out]
                        n174 = call-poly <vilib>:"Write Key.vi"("section"=w290, "error in (no error)"=w280, "value"=w291, "key"=w292, "refnum"=w276) -> ("error out"=w278:errorcluster)  [unwired: 1 in, 5 out]
                        n175 = call-poly <vilib>:"Write Key.vi"("section"=w290, "error in (no error)"=w278, "value"=w288, "key"=w289, "refnum"=w276) -> ("error out"=w282:errorcluster, "refnum out"=w287:T8)  [unwired: 1 in, 4 out]
                        n176 = call "Subvi Event Log.vi"("CustomMessage"=w284) -> ()  [unwired: 1 in]
                        n177 = call <vilib>:"Close Config Data.vi"("error in (no error)"=w282, "refnum"=w287) -> ("error out"=w283:errorcluster)  [unwired: 1 in, 8 out]
                        n178 = call <vilib>:"Simple Error Handler.vi"("error in (no error)"=w283) -> ()  [unwired: 1 in, 8 out]
                      }
                      frame True {
                        # "Load Protocol"
                        n179 = Concatenate Strings("Loading Protocol from " ("string"), w301) -> (w300:string)
                        n180 = call-poly <vilib>:"Read Key.vi"("section"=w323, "error in (no error)"=w299, "default value"=w324, "key"=w324, "refnum"=w308) -> ("value"=w322:string)  [unwired: 1 in, 5 out]
                        n181 = call-poly <vilib>:"Read Key.vi"("section"=w323, "default value"=w321, "key"=w321, "refnum"=w308) -> ("value"=w317:string)  [unwired: 2 in, 5 out]
                        n182 = call-poly <vilib>:"Read Key.vi"("section"=w323, "default value"=w320, "key"=w320, "refnum"=w308) -> ("value"=w316:string)  [unwired: 2 in, 5 out]
                        n183 = call-poly <vilib>:"Read Key.vi"("section"=w323, "default value"=w319, "key"=w319, "refnum"=w308) -> ("value"=w315:string)  [unwired: 2 in, 5 out]
                        n184 = call-poly <vilib>:"Read Key.vi"("section"=w323, "default value"=w318, "key"=w318, "refnum"=w308) -> ("value"=w314:string)  [unwired: 2 in, 5 out]
                        n185 = call <vilib>:"Close Config Data.vi"("refnum"=w308) -> ()  [unwired: 2 in, 9 out]
                        n186 = call "Subvi Event Log.vi"("CustomMessage"=w300) -> ()  [unwired: 1 in]
                        n187 = Unflatten From String(type=w309, binary string=w322) -> (value=w307:T10)  [unwired: 1 in, 4 out]
                        n188 = Unflatten From String(type=w310, binary string=w317) -> (value=w306:T11)  [unwired: 1 in, 4 out]
                        n189 = Unflatten From String(type=w311, binary string=w316) -> (value=w305:T12)  [unwired: 1 in, 4 out]
                        n190 = Unflatten From String(type=w312, binary string=w315) -> (value=w304:cluster{"Lamp Delay":dbl})  [unwired: 1 in, 4 out]
                        n191 = Unflatten From String(type=w313, binary string=w314) -> (value=w303:T13)  [unwired: 1 in, 4 out]
                        n192 = stacked-sequence {
                          tunnel: w307 -> [w331 _ _ _ _]
                          tunnel: w306 -> [_ w343 _ _ _]
                          tunnel: w305 -> [_ _ w351 _ _]
                          tunnel: w304 -> [_ _ _ w353 _]
                          tunnel: w303 -> [_ _ _ _ w359]
                          frame #0 {
                            # "Sectioning Tab"
                            n193 = Unbundle(w331) -> ("PI"=w325:string, "User"=w326:string, "OpSpecimen"=w327:string, "OpSliceThk"=w328:u16, "OpNotes"=w329:string, "Image"=w330:bool)
                            n194 = local write "OpSpecimen"(w327) -> ()
                            n195 = local write "OpSliceThk"(w328) -> ()
                            n196 = local write "OpNotes"(w329) -> ()
                            n197 = local write "Image"(w330) -> ()
                            n198 = local write "User"(w326) -> ()
                            n199 = local write "PI"(w325) -> ()
                          }
                          frame #1 {
                            # "Imaging Tab"
                            n200 = Unbundle(w343) -> ("ImageSkipNum"=w342:i32, "FileNumStart"=w341:i32, "FileNumbering"=w340:enum32{"Continuous", "With Section No."}, "FullFileName"=w338:string, "BaseDir"=w337:string, "ImageRepeatNum"=w339:u32, "BrExpMem"=w336:dbl, "FlExpMem"=w335:dbl, "ImageType"=w334:u16, "IntervalMode"=w333:u16, "ImageInterval"=w332:i32)
                            n201 = local write "ImageSkipNum"(w342) -> ()
                            n202 = local write "FileNumbering"(w340) -> ()
                            n203 = local write "FullFileName"(w338) -> ()
                            n204 = local write "ImageRepeatNum"(w339) -> ()
                            n205 = local write "FileNumStart"(w341) -> ()
                            n206 = local write "BrExpMem"(w336) -> ()
                            n207 = local write "FlExpMem"(w335) -> ()
                            n208 = local write "IntervalMode"(w333) -> ()
                            n209 = local write "ImageType"(w334) -> ()
                            n210 = local write "ImageInterval"(w332) -> ()
                            n211 = local write "BaseDir"(w337) -> ()
                            n212 = global write "ProSCI Global.vi" "gImageInterval"(w332) -> ()
                            n213 = global write "ProSCI Global.vi" "gIntervalMode"(w333) -> ()
                            n214 = global write "ProSCI Global.vi" "gImageType"(w334) -> ()
                            n215 = global write "ProSCI Global.vi" "gBrExpMem"(w336) -> ()
                            n216 = global write "ProSCI Global.vi" "gFlExpMem"(w335) -> ()
                            n217 = global write "ProSCI Global.vi" "gBaseFile"(w338) -> ()
                            n218 = global write "ProSCI Global.vi" "gBaseDir"(w337) -> ()
                          }
                          frame #2 {
                            # "ROI Tab"
                            n219 = Unbundle(w351) -> ("Obj"=w345:u8, "Mag"=w344:u8, "ItemNames"=w350:string[][], "TileXYCoordinates"=w349:i32[][], "TotROI"=w348:i32)
                            n220 = local write "TileXYCoordinates"(w349) -> ()
                            n221 = local write "Obj"(w345) -> ()
                            n222 = local write "Mag"(w344) -> ()
                            n223 = local write "TotROI"(w348) -> ()
                            n224 = property on="ROI List" class="MCListbox (strict)"("Item Names"=w350) -> ()  [unwired: 2 in, 2 out]
                            n225 = global write "ProSCI Global.vi" "gObj"(w345) -> ()
                            n226 = Number To Decimal String(number=w345) -> (decimal integer string=w347:string)  [unwired: 1 out]
                            n227 = Number To Decimal String(number=w344) -> (decimal integer string=w346:string)  [unwired: 1 out]
                            n228 = global write "ProSCI Global.vi" "gMag"(w344) -> ()
                            n229 = property on="Objective" class="CmbBox"("Value"=w347) -> ()  [unwired: 2 in, 2 out]
                            n230 = property on="Magnification" class="CmbBox"("Value"=w346) -> ()  [unwired: 2 in, 2 out]
                          }
                          frame #3 {
                            # "Illumination Tab"
                            n231 = Unbundle(w353) -> ("Lamp Delay"=w352:dbl)
                            n232 = local write "Lamp Delay"(w352) -> ()
                          }
                          frame #4 {
                            # "Maintenance Tab"
                            n233 = Unbundle(w359) -> ("Time Out (sec)"=w358:dbl, "Overlap"=w357:u8, "MinOverlap"=w356:bool, "EProfile"=w355:bool, "Image Delay (sec)"=w354:dbl)
                            n234 = local write "Time Out (sec)"(w358) -> ()
                            n235 = local write "MinOverlap"(w356) -> ()
                            n236 = local write "Overlap"(w357) -> ()
                            n237 = local write "EProfile"(w355) -> ()
                            n238 = local write "Image Delay (sec)"(w354) -> ()
                          }
                        }
                      }
                    }
                    n239 = Strip Path(path=w255) -> (name=w273:string)  [unwired: 1 out]
                    n240 = Concatenate Strings("Pro-SCI - " ("string"), w273) -> (w274:string)
                    n241 = property class="VI"("Front Panel Window:Title"=w274) -> ()  [unwired: 2 in, 2 out]
                  }
                  frame True {
                  }
                }
              }
            }
          }
          frame "Upd_Meta" {
            "UpdateMetadata" <- TRUE
          }
          frame "About" {
            n242 = call "About ProSCI.vi"() -> ()  [unwired: 1 out]
          }
        }
      }
      event "OffsetPx", "OpSliceThk", "Pixel Size": Value Change {
        # "Displacement/micron up"
        n243 = event-data() -> ()  [unwired: 7 out]
        n244 = global read "ProSCI ConfigGlobal.vi" "gCfgMicronPerMicronThickness"() -> (w361:dbl)
        n245 = local read "OpSliceThk"() -> (w372:u16)
        n246 = local read "Pixel Size"() -> (w379:dbl)
        n247 = Equal To 0?(x=w372) -> (x = 0?=w373:bool)
        n248 = Select(t=u16 1, s=w373, f=w372) -> (s? t:f=w370:u16)
        n249 = Multiply(x="OffsetPx", y=w379) -> (x*y=w378:dbl)
        n250 = Multiply(x=w361, y=w370) -> (x*y=w376:dbl)
        n251 = Divide(x=w378, y=w376) -> (x/y=w374:dbl)
        n252 = global read "ProSCI ConfigGlobal.vi" "gCfgMicronPerStep"() -> (w368:dbl)
        n253 = Absolute Value(x=w374) -> (abs(x)=w375:dbl)
        n254 = Round Toward -Infinity(1:w375) -> (0:w377:dbl)
        "OffsetSlice" <- w377
        n255 = Multiply(x=w377, y=w376) -> (x*y=w369:dbl)
        n256 = Divide(x=w369, y=w368) -> (x/y=w367:dbl)
        n257 = Round To Nearest(number=w367) -> (nearest integer value=w366:dbl)
        "AutoXOffset" <- w366
        n258 = Number To Decimal String(number=w366) -> (decimal integer string=w364:string)  [unwired: 1 out]
        n259 = Concatenate Strings("Auto X Offset = ", w364, " motor steps.") -> (w362:string)
        n260 = call "Subvi Event Log.vi"("CustomMessage"=w362) -> ()  [unwired: 1 in]
      }
      event Application Instance Close? {
        n261 = event-data() -> ()  [unwired: 6 out]
        n262 = local read "Current State"() -> (w383:T5)
        n263 = call "Subvi Shutdown ProSCI.vi"("Current State"=w383) -> ("Shutdown"=w381:bool)
        n264 = Not(x=w381) -> (.not. x?=w382:bool)
        n265 = local write "stop"(w381) -> ()
        n266 = event-data("SilentShutdown"=TRUE, "Discard?"=w382) -> ()  [unwired: 1 in, 1 out]
      }
      event "Lamp On": Value Change {
        n267 = event-data() -> ("NewVal"=w385:bool)  [unwired: 6 out]
        n268 = global write "ProSCI Global.vi" "gBrLampOn"(w385) -> ()
      }
      event "Shutter On": Value Change {
        n269 = event-data() -> ("NewVal"=w386:bool)  [unwired: 6 out]
        n270 = global write "ProSCI Global.vi" "gFlLampOn"(w386) -> ()
      }
      event "FlConnectButton": Mouse Up {
        n271 = event-data() -> ()  [unwired: 9 out]
        n272 = flat-sequence {
          frame #0 {
            n273 = call "IScanOpen.vi"("Port"="port 2") -> ("PRIORLib.IScanOut"=w389:refnum<k7>)  [unwired: 2 out]
            n274 = global write "priorlibscanout.vi" "PRIORLib.IScanOut"(w389) -> ()
            "FlConnection" <- TRUE
          }
          frame #1 {
            n275 = call "IFilterOpen.vi"() -> ("PRIORLib.IFilterOut"=w390:refnum<k7>)  [unwired: 2 out]
            n276 = global write "priorlibfilterout.vi" "PRIORLib.IFilterOut"(w390) -> ()
          }
          frame #2 {
            n277 = property on="FlConnectButton" class="Bool (strict)"("Disabled"=2) -> ()  [unwired: 2 in, 2 out]
          }
        }
      }
      event "FlDisonnectButton": Mouse Up {
        n278 = event-data() -> ()  [unwired: 9 out]
        n279 = flat-sequence {
          frame #0 {
            n280 = global read "priorlibscanout.vi" "PRIORLib.IScanOut"() -> (w393:refnum<k7>)
            n281 = property on="FlConnection" class="Bool (strict)"("Value"=FALSE) -> ()  [unwired: 2 in, 2 out]
            n282 = call "IScanClose.vi"("PRIORLib.IScan"=w393) -> ()  [unwired: 2 out]
          }
          frame #1 {
            n283 = property on="FlConnectButton" class="Bool (strict)"("Disabled"=0) -> ()  [unwired: 2 in, 2 out]
          }
        }
      }
      event "BrConnectButton": Mouse Up {
        n284 = event-data() -> ()  [unwired: 9 out]
        n285 = stacked-sequence {
          seq-local: [w395 _] -> [_ w409]
          frame #0 {
            n286 = call "subDCRConnect.vi"() -> ("Firmware Version"=→"BrFWVer":string, "VISA resource name Out"=w395:refnum<visa-resource-name>, "ConnectStatus"=w397:bool)
            "BrConnection" <- w397
            "Br VISA Ref" <- w395
            n287 = call "subDCRStatus.vi"("VISA resource name"=w395) -> ("StatusCode"=→"BrLampStatus":u8)  [unwired: 1 out]
            n288 = Or(x=w397, y=TRUE) -> (x .or. y?=w400:bool)
            n289 = Select(t=2.0, s=w400, f=0.0) -> (s? t:f=w396:dbl)
            n290 = property on="BrConnectButton" class="Bool (strict)"("Disabled"=w396) -> ()  [unwired: 2 in, 2 out]
          }
          frame #1 {
            # "Send Default Intensity Value."
            n291 = Multiply(x=255.0, y="Intensity") -> (x*y=w408:dbl)
            n292 = Divide(x=w408, y=100.0) -> (x/y=w406:dbl)
            n293 = To Long Integer(number=w406) -> (32bit integer=w404:i32)
            n294 = Number To Hexadecimal String(1:i16 2 ("width (-)"), 2:w404) -> (0:w413:string)
            n295 = Concatenate Strings("&ia" ("string"), w413, "\r") -> (w411:string)
            n296 = VISA Write(VISA resource name=w409, write buffer=w411) -> ()  [unwired: 1 in, 3 out]
          }
        }
      }
      event "BrDisonnectButton": Mouse Up {
        # "Note:Closing the serial port allows it to be used by other applications without\nquitting LabVIEW."
        # "Close session to port."
        n297 = event-data() -> ()  [unwired: 9 out]
        n298 = local read "Br VISA Ref"() -> (w419:refnum<visa-resource-name>)
        n299 = VISA Close(VISA resource name=w419) -> (error out=w424:errorcluster)  [unwired: 1 in]
        n300 = call <vilib>:"Simple Error Handler.vi"("error in (no error)"=w424) -> ()  [unwired: 1 in, 8 out]
        n301 = local read "BrConnection"() -> (w418:bool)
        n302 = Or(x=w418, y=TRUE) -> (x .or. y?=w422:bool)
        n303 = Select(t=0.0, s=w422, f=2.0) -> (s? t:f=w417:dbl)
        n304 = local write "BrConnection"(FALSE) -> ()
        n305 = property on="BrConnectButton" class="Bool (strict)"("Disabled"=w417) -> ()  [unwired: 2 in, 2 out]
      }
      event Panel Close? {
        n306 = event-data() -> ()  [unwired: 5 out]
        n307 = local read "Current State"() -> (w425:T5)
        n308 = call "Subvi Shutdown ProSCI.vi"("Current State"=w425) -> ("Shutdown"=w426:bool)
        n309 = local write "stop"(w426) -> ()
        n310 = Not(x=w426) -> (.not. x?=w427:bool)
        n311 = event-data("Discard?"=w427) -> ()  [unwired: 1 in, 1 out]
      }
      event "Intensity": Value Change {
        n312 = event-data() -> ("NewVal"=w429:u8)  [unwired: 6 out]
        n313 = local read "BrConnection"() -> (w428:bool)
        n314 = case shown="True" w428 {
          tunnel: [_ w445] -> w431
          tunnel: [_ w444] -> w430
          tunnel: w429 -> [_ w433]
          frame False {
          }
          frame True {
            n315 = Multiply(x=255.0, y=w433) -> (x*y=w436:dbl)
            n316 = Divide(x=w436, y=u8 100) -> (x/y=w434:dbl)
            n317 = To Long Integer(number=w434) -> (32bit integer=w432:i32)
            n318 = Number To Hexadecimal String(1:i16 2 ("width (-)"), 2:w432) -> (0:w441:string)
            n319 = local read "Br VISA Ref"() -> (w437:refnum<visa-resource-name>)
            n320 = Concatenate Strings("&ia" ("string"), w441, "\r") -> (w439:string)
            n321 = VISA Write(VISA resource name=w437, write buffer=w439) -> (VISA resource name out=w445:refnum<visa-resource-name>, error out=w444:errorcluster)  [unwired: 1 in, 1 out]
          }
        }
      }
      event "RobotStop": Mouse Down {
        # "Kill movement on all axes"
        n322 = event-data() -> ()  [unwired: 9 out]
        n323 = VISA Write(VISA resource name=w446, write buffer="K") -> ()  [unwired: 1 in, 3 out]
      }
      event "FluoExpArray": Value Change {
        n324 = event-data() -> ()  [unwired: 7 out]
        n325 = Array Max & Min(array="FluoExpArray") -> (max value=w450:dbl)  [unwired: 3 out]
        n326 = Not Equal To 0?(x=w450) -> (x != 0?=w449:bool)
        n327 = global write "ProSCI Global.vi" "gMultiFluoExp"(w449) -> ()
        n328 = case shown="True" w449 {
          tunnel: "FluoExpArray" -> [_ w456]
          frame False {
          }
          frame True {
            n329 = global write "ProSCI Global.vi" "gFluoExpArray"(w456) -> ()
            n330 = for {
              tunnel: w456 -> [w462] mode=indexing
              shift-right: [w460] -> w455
              shift-left: 0 -> [w459]
              n331 = Not Equal To 0?(x=w462) -> (x != 0?=w461:bool)
              n332 = Increment(x=w459) -> (x+1=w458:i32)
              n333 = Select(t=w458, s=w461, f=w459) -> (s? t:f=w460:i32)
            }
            n334 = Number To Decimal String(number=w455) -> (decimal integer string=w454:string)  [unwired: 1 out]
            n335 = Concatenate Strings("Additional ", w454, " Fluo exposures entered.") -> (w451:string)
            n336 = call "Subvi Event Log.vi"("CustomMessage"=w451) -> ()  [unwired: 1 in]
          }
        }
      }
      event "SampleThk": Value Change {
        n337 = event-data() -> ()  [unwired: 7 out]
        n338 = local read "OpSliceThk"() -> (w465:u16)
        n339 = Multiply(x="SampleThk", y=u32 1000) -> (x*y=w466:u32)
        n340 = Divide(x=w466, y=w465) -> (x/y=w464:dbl)
        n341 = Round Toward +Infinity(x=w464) -> (ceil(x): smallest int >= x=w463:dbl)
        n342 = local write "Total Cuts"(w463) -> ()
      }
      event "ROI List": Value Change {
        n343 = event-data() -> ()  [unwired: 7 out]
        n344 = stacked-sequence {
          frame #0 {
            w469 = FALSE ("IO Cut Comp")
            n345 = property on="LeftEdge" class="Bool"("Visible"=w469) -> ()  [unwired: 2 in, 2 out]
            n346 = property on="RightEdge" class="Bool"("Visible"=w469) -> ()  [unwired: 2 in, 2 out]
            n347 = property on="TopEdge" class="Bool"("Visible"=w469) -> ()  [unwired: 2 in, 2 out]
            n348 = property on="BotEdge" class="Bool"("Visible"=w469) -> ()  [unwired: 2 in, 2 out]
            n349 = local read "RobotOnline"() -> (w470:bool)
            n350 = case shown="True" w470 {
              frame False {
              }
              frame True {
                n351 = property on="Tile ROI" class="Bool"("Disabled"=u8 0) -> ()  [unwired: 2 in, 2 out]
              }
            }
          }
        }
      }
    }
  }
  n352 = while {
    tunnel: w9 -> [w472]
    stop <- w488 stop-if-true
    n353 = local read "Mag"() -> (w486:u8)
    n354 = local read "Obj"() -> (w487:u8)
    n355 = local read "RobotIndexed"() -> (w479:bool)
    n356 = Not(x=w479) -> (.not. x?=w480:bool)
    n357 = And(x="RobotIdx", y=w480) -> (x .and. y?=w478:bool)
    n358 = stacked-sequence {
      tunnel: w486 -> [_ _ _ w612 w624]
      tunnel: w487 -> [_ _ _ w611 w623]
      tunnel: w472 -> [w588 w597 w604 w610 w622]
      frame #0 {
        n359 = case shown="False" "RobotJog" {
          tunnel: w588 -> [_ w590]
          frame False {
          }
          frame True {
            n360 = stacked-sequence {
              tunnel: w590 -> [_ w592 _]
              frame #0 {
                n361 = local write "Robot State"(T15."Jog" ("Robot State")) -> ()
              }
              frame #1 {
                n362 = call "newsubvi Robot Jog Control.vi"("VISA In"=w592) -> ()  [unwired: 1 out]
              }
              frame #2 {
                n363 = local read "RobotIndexed"() -> (w596:bool)
                n364 = Select(t=T15."Idle" ("Robot State"), s=w596, f=T16."Not Indexed" ("Robot State")) -> (s? t:f=w593:T16)
                n365 = local write "Robot State"(w593) -> ()
              }
            }
          }
        }
      }
      frame #1 {
        n366 = case shown="False" "RobotIndex" {
          tunnel: w597 -> [_ w599]
          frame False {
          }
          frame True {
            n367 = stacked-sequence {
              tunnel: w599 -> [_ w601 _]
              frame #0 {
                n368 = local write "Robot State"(T15."Indexing" ("Robot State")) -> ()
              }
              frame #1 {
                n369 = call "newsubvi Robot Index to Zero.vi"("VISA In"=w601) -> ()  [unwired: 2 out]
              }
              frame #2 {
                n370 = local write "Robot State"(T15."Idle" ("Robot State")) -> ()
                "RobotIndexed" <- TRUE ("RobotIndexed")
              }
            }
          }
        }
      }
      frame #2 {
        n371 = case shown="False" "RobotPark" {
          tunnel: w604 -> [_ w606]
          frame False {
          }
          frame True {
            n372 = stacked-sequence {
              tunnel: w606 -> [_ w608 _]
              frame #0 {
                n373 = local write "Robot State"(T15."Parking" ("Robot State")) -> ()
              }
              frame #1 {
                n374 = call "newsubvi Robot GoTo Park.vi"("VISA In"=w608) -> ()  [unwired: 2 out]
              }
              frame #2 {
                n375 = local write "Robot State"(T15."Idle" ("Robot State")) -> ()
              }
            }
          }
        }
      }
      frame #3 {
        n376 = case shown="False" "RobotImage" {
          tunnel: w612 -> [_ w616]
          tunnel: w611 -> [_ w615]
          tunnel: w610 -> [_ w614]
          frame False {
          }
          frame True {
            n377 = stacked-sequence {
              tunnel: w616 -> [_ w620 _]
              tunnel: w615 -> [_ w619 _]
              tunnel: w614 -> [_ w618 _]
              frame #0 {
                n378 = local write "Robot State"(T15."Moving to Image" ("Robot State")) -> ()
              }
              frame #1 {
                n379 = call "newsubvi Robot GoTo Image.vi"("Magnification"=w620, "Objective"=w619, "VISA In"=w618) -> ()  [unwired: 2 out]
              }
              frame #2 {
                n380 = local write "Robot State"(T15."Idle" ("Robot State")) -> ()
              }
            }
          }
        }
      }
      frame #4 {
        n381 = case shown="True" "RobotFocus" {
          tunnel: w624 -> [_ w628]
          tunnel: w623 -> [_ w627]
          tunnel: w622 -> [_ w626]
          frame False {
          }
          frame True {
            n382 = stacked-sequence {
              tunnel: w628 -> [_ w632 _]
              tunnel: w627 -> [_ w631 _]
              tunnel: w626 -> [_ w630 _]
              frame #0 {
                n383 = local write "Robot State"(T15."Focusing" ("Robot State")) -> ()
              }
              frame #1 {
                n384 = call "newsubvi Robot GoTo Focus.vi"("Magnification"=w632, "Objective"=w631, "VISA In"=w630) -> ()  [unwired: 2 out]
              }
              frame #2 {
                n385 = local write "Robot State"(T15."Idle" ("Robot State")) -> ()
              }
            }
          }
        }
      }
    }
    n386 = Wait (ms)(milliseconds to wait=u32 25) -> ()  [unwired: 1 out]
    n387 = case shown="False" "Image ROI" {
      tunnel: [FALSE ("Safe") w491] -> w476
      frame False {
      }
      frame True {
        n388 = call "newSubvi Safety Check.vi"("SafetyCheck"=T14."Exposure") -> ("Safe"=w491:bool)  [unwired: 4 in, 2 out]
        n389 = case shown="True" w491 {
          frame False {
          }
          frame True {
            n390 = local read "ImageType"() -> (w493:u16)
            n391 = call "Subvi Setup Lamp And Exposure.vi"("PassImageType"=w493) -> ()
          }
        }
      }
    }
    n392 = case shown="False" w478 {
      frame False {
      }
      frame True {
        n393 = Two Button Dialog(message="CAUTION!!\nThis will bypass Indexing Sequence and put system in Indexed State.\nShould only be used if Velmex Black Box has not been switched off\nsince last Indexing operation but ProSci has been restarted.\nCancel if not sure.\n\nContinue with operation?", 2:"Yes" ("T button name (\"OK\")")) -> (T button?=w582:bool)  [unwired: 1 out]
        n394 = case shown="True" w582 {
          frame False {
          }
          frame True {
            n395 = call "Subvi Event Log.vi"("EventNum"=u32 19) -> ()  [unwired: 1 in]
            n396 = local write "RobotIndexed"(TRUE ("RobotIndexed")) -> ()
            n397 = local write "Robot State"(T3."Idle" ("Robot State")) -> ()
          }
        }
      }
    }
    n398 = local read "SecNumInFile"() -> (w474:u32)
    n399 = local read "FileNumStart"() -> (w475:i32)
    n400 = local read "ImageNow"() -> (w485:bool)
    n401 = property on="ROI List" class="MCListbox (strict)"() -> ("Item Names"=w483:string[][], "Value"=w482:i32)  [unwired: 2 in, 2 out]
    n402 = Select(t=w475, s=w476, f=w474) -> (s? t:f=w473:u32)
    n403 = Or(x=w476, y=w485) -> (x .or. y?=w484:bool)
    n404 = stacked-sequence {
      tunnel: w483 -> [w496 w521]
      tunnel: w482 -> [w495 w520]
      tunnel: w472 -> [w494 w517]
      frame #0 {
        n405 = case shown="False" "MoveTo ROI" {
          tunnel: w496 -> [_ w501]
          tunnel: w495 -> [_ w500]
          tunnel: w494 -> [_ w498]
          frame False {
          }
          frame True {
            n406 = flat-sequence {
              tunnel: w501 -> [w506]
              tunnel: w500 -> [w505]
              tunnel: [w503] -> w499
              tunnel: w499 -> [w514]
              tunnel: w498 -> [w507]
              frame #0 {
                n407 = call "subvi Robot Extract ROI Info.vi"("ROIListBoxIn"=w506, "Selection"=w505) -> ("XYListOffset"=w503:u32)  [unwired: 3 out]
                n408 = local write "Robot State"(T15."Moving to ROI" ("Robot State")) -> ()
                n409 = local write "MoveTo ROI"(FALSE) -> ()
              }
              frame #1 {
                n410 = local read "TileXYCoordinates"() -> (w515:i32[][])
                n411 = Index Array(array=w515, index (row)=w514) -> (element=w513:i32[])  [unwired: 1 in]
                n412 = Index Array(array=w513, index=0) -> (element=w510:i32)
                n413 = Index Array(array=w513, index=1) -> (element=w509:i32)
                n414 = call "newsubvi Robot GoTo XY.vi"("GoToY"=w509, "GoToX"=w510, "Slow Speed"=TRUE ("Add Offset"), "VISA In"=w507) -> ()  [unwired: 2 out]
              }
              frame #2 {
                n415 = local write "Robot State"(T15."Idle" ("Robot State")) -> ()
              }
            }
          }
        }
      }
      frame #1 {
        n416 = Or(x="StoreGlobalOffset", y="ClearGlobalOffset") -> (x .or. y?=w522:bool)
        n417 = case shown="False" w522 {
          tunnel: w521 -> [_ w528]
          tunnel: w520 -> [_ w527]
          tunnel: "StoreGlobalOffset" -> [_ w525]
          tunnel: "ClearGlobalOffset" -> [_ w524]
          tunnel: w517 -> [_ w523]
          frame False {
          }
          frame True {
            n418 = local read "TileXYCoordinates"() -> (w526:i32[][])
            n419 = stacked-sequence {
              tunnel: w528 -> [w535 _ _ _]
              tunnel: w527 -> [w534 _ _ _]
              tunnel: w526 -> [w533 w557 _ _]
              tunnel: w525 -> [w532 w560 _ w565]
              tunnel: w524 -> [_ _ w563 _]
              tunnel: w523 -> [w529 _ _ _]
              frame #0 {
                n420 = case shown="True" w532 {
                  tunnel: w535 -> [_ w551]
                  tunnel: w534 -> [_ w550]
                  tunnel: w533 -> [_ w549]
                  tunnel: [u32 21 ("EventNum") u32 20 ("EventNum")] -> w531
                  tunnel: [FALSE TRUE] -> w530
                  tunnel: w529 -> [_ w538]
                  frame False {
                  }
                  frame True {
                    # "Calculate Offset"
                    n421 = call "subvi Robot Extract ROI Info.vi"("ROIListBoxIn"=w551, "Selection"=w550) -> ("XYListOffset"=w548:u32)  [unwired: 3 out]
                    n422 = call "newsubvi Robot Get XY.vi"("VISA In"=w538) -> ("XPosition"=w545:i32, "YPosition"=w546:i32)  [unwired: 2 out]
                    n423 = Index Array(array=w549, index (row)=w548) -> (element=w547:i32[])  [unwired: 1 in]
                    n424 = Index Array(array=w547, index=0) -> (element=w544:i32)
                    n425 = Subtract(x=w545, y=w544) -> (x-y=w542:i32)
                    n426 = Index Array(array=w547, index=1) -> (element=w543:i32)
                    n427 = Subtract(x=w546, y=w543) -> (x-y=w541:i32)
                    n428 = global write "ProSCI Global.vi" "gGlobalOffsetY"(w541) -> ()
                    n429 = global write "ProSCI Global.vi" "gGlobalOffsetX"(w542) -> ()
                  }
                }
                "OffsetPresent" <- w530
                n430 = call "Subvi Event Log.vi"("EventNum"=w531) -> ()  [unwired: 1 in]
              }
              frame #1 {
                # "Update XY Coordinate Array - if store then add offset, if clear then subtract"
                n431 = global read "ProSCI Global.vi" "gGlobalOffsetX"() -> (w562:i32)
                n432 = Negate(x=w562) -> (-x=w561:i32)
                n433 = global read "ProSCI Global.vi" "gGlobalOffsetY"() -> (w558:i32)
                n434 = Negate(x=w558) -> (-x=w559:i32)
                n435 = Select(t=w562, s=w560, f=w561) -> (s? t:f=w556:i32)
                n436 = Select(t=w558, s=w560, f=w559) -> (s? t:f=w555:i32)
                n437 = call "Subvi Add Offset to XY Coordinates.vi"("YOffsetIn"=w555, "XOffsetIn"=w556, "TileXYCoordinatesIn"=w557) -> ("TileXYCoordinatesOut"=w554:i32[][])
                n438 = local write "TileXYCoordinates"(w554) -> ()
              }
              frame #2 {
                # "If Clear was selected,\nset offsets to zero"
                n439 = case shown="True" w563 {
                  frame False {
                  }
                  frame True {
                    w564 = 0
                    n440 = global write "ProSCI Global.vi" "gGlobalOffsetY"(w564) -> ()
                    n441 = global write "ProSCI Global.vi" "gGlobalOffsetX"(w564) -> ()
                  }
                }
              }
              frame #3 {
                n442 = stacked-sequence {
                  tunnel: w565 -> [_ w570]
                  frame #0 {
                    # "Store Offset in Metadata File"
                    n443 = global read "ProSCI Global.vi" "gGlobalOffsetY"() -> (w566:i32)
                    n444 = global read "ProSCI Global.vi" "gGlobalOffsetX"() -> (w567:i32)
                    n445 = local read "FileNumStart"() -> (w568:i32)
                    n446 = call "Subvi Write Metadata.vi"("YOffsetIn"=w566, "XOffsetIn"=w567, "Next Cut"=w568, "Store Offset (F)"=TRUE) -> ()  [unwired: 4 in]
                  }
                  frame #1 {
                    n447 = case shown="True" w570 {
                      frame False {
                      }
                      frame True {
                        n448 = One Button Dialog(message="You should perform File|Save Protocol\nto store offset values for later use.") -> ()  [unwired: 2 out]
                      }
                    }
                  }
                }
              }
            }
          }
        }
      }
    }
    n449 = case shown="False" w484 {
      tunnel: w483 -> [_ w577]
      tunnel: w482 -> [_ w576]
      tunnel: w476 -> [_ w575]
      tunnel: w473 -> [_ w573]
      tunnel: w472 -> [_ _]
      frame False {
      }
      frame True {
        n450 = local read "OpSliceThk"() -> (w572:u16)
        n451 = local read "FullFileName"() -> (w581:string)
        n452 = call "Subvi SetFileName.vi"("Thickness"=w572, "SectionNumInFile"=w573, "BaseFile"=w581) -> ("ImageFile"=w580:string)
        n453 = call "newSubvi MultiROI Image.vi"("ROISelected"=w576, "Snap"=w575, "ImageRepeatNum"="ImageRepeatNum", "ROIListBoxIn"=w577, "BaseFileName"=w580) -> ("ImagingDone"=→"Imaging Done":bool)  [unwired: 2 in]
        n454 = local write "ImageNow"(FALSE) -> ()
      }
    }
    n455 = local read "stop"() -> (w488:bool)
  }
  n456 = while {
    shift-right: [w667] -> _
    shift-left: T5."Emergency Off" -> [w668]
    shift-right: [w642] -> _
    shift-left: 0 -> [w675]
    shift-right: [w671] -> _
    shift-left: 0 -> [w672]
    shift-right: [w674] -> _
    shift-left: 0 -> [w673]
    shift-right: [w661] -> _
    shift-left: 0 -> [w663]
    shift-right: [w641] -> _
    shift-left: 0 -> [w640]
    tunnel: w16 -> [w638]
    stop <- w670 stop-if-true
    w662 = u32 80 ("millisecond multiple")
    # "Load Protocol Enabled only in Idle State"
    # "Cut Buttons enabled\nonly in Idle State"
    # "Sequence Cut Reset here"
    # "State Specific Actions down here"
    # "Waits for 80 ms\nfor front panel activity"
    n457 = local read "Current State"() -> (w652:T5)
    n458 = local read "IO Cut Comp"() -> (w634:bool)
    "CutCompXition" <- w634
    n459 = local read "Total Cuts"() -> (w649:u32)
    n460 = local read "IO EStop?"() -> (w669:bool)
    n461 = local read "Sequence Cut"() -> (w657:bool)
    n462 = Not Equal To 0?(x=w649) -> (x != 0?=w648:bool)
    n463 = Select(t=0, s=w657, f=2) -> (s? t:f=w658:i32)
    n464 = Equal?(x=w652, y=T5."Idle") -> (x = y?=w639:bool)
    n465 = case shown="\"Illumination\"" "Tab Control" {
      tunnel: "Robot VISA Ref" -> [_ _ _ w709 w762]
      frame "Sectioning", Default {
      }
      frame "Imaging" {
        n466 = Or(x="SetFile Button", y="Capture Single Image") -> (x .or. y?=w691:bool)
        n467 = case shown="True" w691 {
          tunnel: "SetFile Button" -> [_ w704]
          tunnel: "Capture Single Image" -> [_ w699]
          frame False {
          }
          frame True {
            n468 = local read "OpSpecimen"() -> (w703:string)
            n469 = Select(t=w703, s=w704, f="") -> (s? t:f=w702:string)
            n470 = call "Subvi Select Directory.vi"("Prompt"=w702) -> ("FullFileName"=w697:string, "Dir Name"=→"BaseDir":string, "Cancelled"=w700:bool)
            "FullFileName" <- w697
            n471 = Not(x=w700) -> (.not. x?=w701:bool)
            n472 = And(x=w701, y=w699) -> (x .and. y?=w698:bool)
            n473 = case shown="True" w698 {
              tunnel: w697 -> [_ w707]
              frame False {
              }
              frame True {
                n474 = call "Subvi Acquire Image.vi"("ImgFile"=w707) -> ()  [unwired: 2 out]
              }
            }
          }
        }
        n475 = stacked-sequence {
          frame #0 {
            n476 = global read "ProSCI Global.vi" "gBrExpMem"() -> (→"BrExpMem":dbl)
          }
          frame #1 {
            n477 = global read "ProSCI Global.vi" "gFlExpMem"() -> (→"FlExpMem":dbl)
          }
          frame #2 {
            n478 = global write "ProSCI Global.vi" "gImageType"("ImageType") -> ()
            n479 = global write "ProSCI Global.vi" "gIntervalMode"("IntervalMode") -> ()
            n480 = global write "ProSCI Global.vi" "gImageInterval"("ImageInterval") -> ()
          }
        }
      }
      frame "Illumination" {
        n481 = global read "ProSCI Global.vi" "gBrLampOn"() -> (w708:bool)
        n482 = local write "Lamp On"(w708) -> ()
      }
      frame "Maintenance" {
        n483 = stacked-sequence {
          tunnel: w709 -> [w710 _]
          frame #0 {
            n484 = local read "RobotOnline"() -> (w713:bool)
            n485 = local read "RobotIndexed"() -> (w712:bool)
            n486 = And(x=w713, y=w712) -> (x .and. y?=w711:bool)
            n487 = case shown="True" w711 {
              tunnel: [2 0] -> w714
              tunnel: w710 -> [_ w716]
              frame False {
              }
              frame True {
                n488 = case shown="True" "SaveFocusData" {
                  tunnel: w716 -> [_ w719]
                  frame False {
                  }
                  frame True {
                    n489 = flat-sequence {
                      tunnel: w719 -> [w721]
                      tunnel: [w722] -> w720
                      tunnel: w720 -> [w726]
                      frame #0 {
                        n490 = call "subvi Robot Get Motor Position.vi"("VISA In"=w721, "Motor Number"=3) -> ("Motor Position"=w724:string)  [unwired: 3 out]
                        n491 = Decimal String To Number(string=w724) -> (number=w723:i32)  [unwired: 3 out]
                        n492 = Absolute Value(x=w723) -> (abs(x)=w722:i32)
                      }
                      frame #1 {
                        w729 = "Robot" ("section")
                        n493 = String To Path(string="C:\\Program Files\\ProSCI\\ProSciSettings.ini") -> (path=w741:path)
                        n494 = call <vilib>:"Open Config Data (compatibility).vi"("create file if necessary (T)"=FALSE ("create file if necessary? (T)"), "configuration file path"=w741) -> ("error out"=w736:errorcluster, "refnum"=w738:T8)  [unwired: 7 in, 1 out]
                        n495 = call-poly <vilib>:"Write Key.vi"("section"=w729, "error in (no error)"=w736, "value"=w726, "key"="FocusZPos", "refnum"=w738) -> ("error out"=w734:errorcluster, "refnum out"=w735:T8)  [unwired: 5 out]
                        n496 = local read "Obj"() -> (w732:u8)
                        n497 = call-poly <vilib>:"Write Key.vi"("section"=w729, "error in (no error)"=w734, "value"=w732, "key"="FocusObj", "refnum"=w735) -> ("error out"=w730:errorcluster, "refnum out"=w731:T8)  [unwired: 5 out]
                        n498 = local read "Mag"() -> (w727:u8)
                        n499 = call-poly <vilib>:"Write Key.vi"("section"=w729, "error in (no error)"=w730, "value"=w727, "key"="FocusMag", "refnum"=w731) -> ("error out"=w743:errorcluster, "refnum out"=w744:T8)  [unwired: 5 out]
                        n500 = call <vilib>:"Close Config Data.vi"("error in (no error)"=w743, "write file if changed (T)"=TRUE ("write configuration file? (T)"), "refnum"=w744) -> ()  [unwired: 9 out]
                      }
                    }
                  }
                }
              }
            }
            n501 = property on="SaveFocusData" class="Bool"("Disabled"=w714) -> ()  [unwired: 2 in, 2 out]
          }
          frame #1 {
            n502 = case shown="True" "ResetKnife" {
              frame False {
              }
              frame True {
                n503 = local read "KnifeTime"() -> (w761:i32)
                n504 = call "Subvi Event Log.vi"("EventNum"=u32 9) -> ()  [unwired: 1 in]
                n505 = Negate(x=w761) -> (-x=w760:i32)
                n506 = local write "KnifeBase"(w760) -> ()
              }
            }
            n507 = case shown="True" "ResetLub" {
              frame False {
              }
              frame True {
                n508 = local read "LubTime"() -> (w758:i32)
                n509 = Negate(x=w758) -> (-x=w757:i32)
                n510 = call "Subvi Event Log.vi"("EventNum"=u32 10) -> ()  [unwired: 1 in]
                n511 = local write "LubBase"(w757) -> ()
              }
            }
            n512 = local read "TotalSessionCuts"() -> (w747:u32)
            n513 = local read "KnifeBase"() -> (w751:i32)
            n514 = local read "LubBase"() -> (w748:i32)
            n515 = Add(x=w751, y=w747) -> (x+y=w746:u32)
            "KnifeTime" <- w746
            n516 = Add(x=w748, y=w747) -> (x+y=w745:u32)
            "LubTime" <- w745
            n517 = local read "KnifeSetTime"() -> (w750:u32)
            n518 = local read "LubSetTime"() -> (w753:u32)
            n519 = Greater?(x=w746, y=w750) -> (0:→"Change Knife":bool)
            n520 = Greater?(x=w745, y=w753) -> (0:→"Lubricate":bool)
            n521 = global write "ProSCI Global.vi" "gKnifeRun"(w746) -> ()
            n522 = global write "ProSCI Global.vi" "gLubRun"(w745) -> ()
          }
        }
      }
      frame "ROI/Tile" {
        n523 = Decimal String To Number(string="Magnification") -> (number=w763:i32)  [unwired: 3 out]
        "Mag" <- w763
        n524 = Decimal String To Number(string="Objective") -> (number=w764:i32)  [unwired: 3 out]
        "Obj" <- w764
        n525 = local read "EdgeMarker"() -> (w767:u8)
        n526 = global write "ProSCI Global.vi" "gMag"(w763) -> ()
        n527 = property on="ROI List" class="MCListbox (strict)"() -> ("Item Names"=w769:string[][])  [unwired: 2 in, 2 out]
        n528 = global write "ProSCI Global.vi" "gObj"(w764) -> ()
        n529 = call <vilib>:"Trim Whitespace.vi"("string"="ROIName") -> ("trimmed string"=w765:string)  [unwired: 1 in]
        n530 = stacked-sequence {
          tunnel: w769 -> [_ _ w853 w882 w895 w909 _ _ w977 _]
          tunnel: w765 -> [_ _ w852 _ w893 _ _ _ _ _]
          tunnel: "ROI List" -> [_ _ _ w881 w894 w908 _ _ w976 _]
          tunnel: w767 -> [_ _ _ _ _ _ w935 w956 w981 _]
          tunnel: w764 -> [_ _ _ _ _ _ _ _ w979 w1064]
          tunnel: w763 -> [_ _ _ _ _ _ _ _ w978 w1063]
          tunnel: w762 -> [w772 _ w851 _ _ _ w934 w955 _ _]
          frame #0 {
            n531 = case shown="True" "RobotConnect" {
              tunnel: w772 -> [_ w785]
              frame False {
              }
              frame True {
                n532 = stacked-sequence {
                  tunnel: w785 -> [w786 _]
                  frame #0 {
                    n533 = call-poly "VISA Configure Serial Port"("VISA resource name"=w786) -> ("VISA resource name out"=w789:refnum<visa-resource-name>, "error out"=w788:errorcluster)  [unwired: 5 in, 8 out]
                    n534 = VISA Write(VISA resource name=w789, write buffer="F", error in (no error)=w788) -> ()  [unwired: 3 out]
                  }
                  frame #1 {
                    n535 = case shown="True" "Case Constant\n(See Context Help)" {
                      frame False {
                      }
                      frame True {
                        n536 = property on="RobotConnect" class="Bool"("Disabled"=u8 2) -> ()  [unwired: 2 in, 2 out]
                        n537 = local write "Robot State"(T3."Not Indexed" ("Robot State")) -> ()
                        n538 = property on="RobotDisConnect" class="Bool"("Disabled"=u8 0) -> ()  [unwired: 2 in, 2 out]
                      }
                    }
                    "RobotOnline" <- "Case Constant\n(See Context Help)"
                  }
                }
              }
            }
            n539 = case shown="True" "RobotDisConnect" {
              tunnel: w772 -> [_ w775]
              frame False {
              }
              frame True {
                n540 = stacked-sequence {
                  tunnel: w775 -> [w776 _]
                  frame #0 {
                    n541 = VISA Write(VISA resource name=w776, write buffer="Q") -> (VISA resource name out=w778:refnum<visa-resource-name>, error out=w777:errorcluster)  [unwired: 1 in, 1 out]
                    n542 = VISA Close(VISA resource name=w778, error in (no error)=w777) -> ()  [unwired: 1 out]
                  }
                  frame #1 {
                    n543 = local write "RobotOnline"("Case Constant\n(See Context Help) 2") -> ()
                    n544 = case shown="False" "Case Constant\n(See Context Help) 2" {
                      frame False {
                        n545 = property on="RobotConnect" class="Bool"("Disabled"=u8 0) -> ()  [unwired: 2 in, 2 out]
                        n546 = local write "Robot State"(T3."Offline" ("Robot State")) -> ()
                        n547 = property on="RobotDisConnect" class="Bool"("Disabled"=u8 2) -> ()  [unwired: 2 in, 2 out]
                        n548 = local write "RobotIndexed"(FALSE ("IO Cut Comp")) -> ()
                      }
                      frame True {
                      }
                    }
                  }
                }
              }
            }
          }
          frame #1 {
            # "Temporary"
            n549 = case shown="False" "Case Constant\n(See Context Help) 3" {
              frame False {
                n550 = stacked-sequence {
                  frame #0 {
                    w796 = 0 ("t")
                    w797 = 2
                    w800 = u8 0 ("Disabled")
                    n551 = property on="Objective" class="CmbBox"("Disabled"=w800) -> ()  [unwired: 2 in, 2 out]
                    n552 = property on="Magnification" class="CmbBox"("Disabled"=w800) -> ()  [unwired: 2 in, 2 out]
                    n553 = property on="ROI List" class="MCListbox (strict)"("Disabled"=w800) -> ()  [unwired: 2 in, 2 out]
                    n554 = local read "RobotOnline"() -> (w799:bool)
                    n555 = Select(t=w797, s=w799, f=w796) -> (s? t:f=w798:i32)
                    n556 = Select(t=w796, s=w799, f=w797) -> (s? t:f=w795:i32)
                    n557 = property on="RobotConnect" class="Bool"("Disabled"=w798) -> ()  [unwired: 2 in, 2 out]
                    n558 = property on="RobotDisConnect" class="Bool"("Disabled"=w795) -> ()  [unwired: 2 in, 2 out]
                  }
                  frame #1 {
                    n559 = local read "Robot State"() -> (w811:T3)
                    n560 = Equal?(x=w811, y=T3."Offline" ("Robot State")) -> (x = y?=w808:bool)
                    n561 = Equal?(x=T16."Not Indexed" ("Robot State"), y=w811) -> (x = y?=w809:bool)
                    n562 = Equal?(x=w811, y=T15."Idle" ("Robot State")) -> (x = y?=w815:bool)
                    n563 = Or(x=w808, y=w809) -> (x .or. y?=w803:bool)
                    n564 = Or(x=w809, y=w815) -> (x .or. y?=w822:bool)
                    n565 = Select(t=u8 0 ("Disabled"), s=w822, f=u8 2 ("Disabled")) -> (s? t:f=w819:u8)
                    n566 = Select(t=u8 0 ("Disabled"), s=w809, f=u8 2 ("Disabled")) -> (s? t:f=w816:u8)
                    n567 = Select(t=u8 0 ("Disabled"), s=w815, f=u8 2 ("Disabled")) -> (s? t:f=w827:u8)
                    n568 = property on="RobotIndex" class="Bool"("Disabled"=w816) -> ()  [unwired: 2 in, 2 out]
                    n569 = property on="RobotJog" class="Bool"("Disabled"=w819) -> ()  [unwired: 2 in, 2 out]
                    n570 = property on="RobotPark" class="Bool"("Disabled"=w827) -> ()  [unwired: 2 in, 2 out]
                    n571 = property on="MoveTo ROI" class="Bool (strict)"("Disabled"=w827) -> ()  [unwired: 2 in, 2 out]
                    n572 = property on="RobotImage" class="Bool"("Disabled"=w827) -> ()  [unwired: 2 in, 2 out]
                    n573 = property on="RobotFocus" class="Bool"("Disabled"=w827) -> ()  [unwired: 2 in, 2 out]
                    n574 = case shown="True" w803 {
                      frame False {
                      }
                      frame True {
                        n575 = property on="Tile ROI" class="Bool"("Disabled"=u8 2) -> ()  [unwired: 2 in, 2 out]
                      }
                    }
                    n576 = local read "TotROI"() -> (w802:i32)
                    n577 = Equal To 0?(x=w802) -> (x = 0?=w807:bool)
                    n578 = Or(x=w803, y=w807) -> (x .or. y?=w804:bool)
                    n579 = Select(t=u8 2 ("Disabled"), s=w803, f=u8 0 ("Disabled")) -> (s? t:f=w812:u8)
                    n580 = Select(t=u8 2 ("Disabled"), s=w804, f=u8 0 ("Disabled")) -> (s? t:f=w801:u8)
                    n581 = property on="Add ROI" class="Bool"("Disabled"=w812) -> ()  [unwired: 2 in, 2 out]
                    n582 = property on="Rename ROI" class="Bool"("Disabled"=w812) -> ()  [unwired: 2 in, 2 out]
                    n583 = property on="Delete ROI" class="Bool"("Disabled"=w812) -> ()  [unwired: 2 in, 2 out]
                    n584 = property on="Image ROI" class="Bool"("Disabled"=w801) -> ()  [unwired: 2 in, 2 out]
                  }
                  frame #2 {
                    n585 = local read "Sequence Cut"() -> (w843:bool)
                    n586 = local read "OffsetPresent"() -> (w842:bool)
                    n587 = local read "RobotIndexed"() -> (w831:bool)
                    n588 = local read "TotROI"() -> (w829:i32)
                    n589 = Not Equal To 0?(x=w829) -> (x != 0?=w832:bool)
                    n590 = Not(x=w843) -> (.not. x?=w837:bool)
                    n591 = And(x=w831, y=w832) -> (x .and. y?=w830:bool)
                    n592 = And(x=w842, y=w837) -> (x .and. y?=w841:bool)
                    n593 = And(x=w837, y=w830) -> (x .and. y?=w834:bool)
                    n594 = Select(t=0, s=w841, f=2) -> (s? t:f=w838:i32)
                    n595 = Select(t=0, s=w834, f=2) -> (s? t:f=w833:i32)
                    n596 = property on="ClearGlobalOffset" class="Bool"("Disabled"=w838) -> ()  [unwired: 2 in, 2 out]
                    n597 = property on="StoreGlobalOffset" class="Bool"("Disabled"=w833) -> ()  [unwired: 2 in, 2 out]
                  }
                }
              }
              frame True {
                n598 = flat-sequence {
                  frame #0 {
                    # "Sequence On - Disable ROI Tab"
                    n599 = property on="Tab Control" class="TabCtl (strict)"() -> ("Pages"=w844:refnum<vi>[])  [unwired: 2 in, 2 out]
                    n600 = Index Array(array=w844, index=2) -> (element=w846:refnum<vi>)
                    n601 = property class="Page"(reference=w846) -> ("Controls on Page[]"=w845:refnum<vi>[])  [unwired: 1 in, 2 out]
                    n602 = for {
                      tunnel: w845 -> [w849] mode=indexing
                      n603 = property class="Ctl"(reference=w849, "Disabled"=u8 2) -> ()  [unwired: 1 in, 2 out]
                    }
                  }
                  frame #1 {
                    # "Should always be able\nto stop"
                    n604 = property on="RobotStop" class="Bool"("Disabled"=u8 0) -> ()  [unwired: 2 in, 2 out]
                  }
                }
              }
            }
          }
          frame #2 {
            n605 = case shown="True" "Add ROI" {
              tunnel: w853 -> [_ w859]
              tunnel: w852 -> [_ w858]
              tunnel: w851 -> [_ w855]
              frame False {
              }
              frame True {
                # "ROI Name\nNot Blank"
                n606 = String Length(string=w858) -> (length=w857:i32)
                n607 = Not Equal To 0?(x=w857) -> (x != 0?=w856:bool)
                n608 = case shown="True" w856 {
                  tunnel: w859 -> [_ w870]
                  tunnel: w858 -> [_ w869]
                  tunnel: w855 -> [_ w861]
                  frame False {
                    n609 = call "Subvi Event Log.vi"("EventNum"=u32 4) -> ()  [unwired: 1 in]
                  }
                  frame True {
                    w877 = i32[] [] ("TempXYArray")
                    # "Highlight Last ROI Added"
                    n610 = local write "TempXYArray"(w877) -> ()
                    n611 = call "newsubvi Robot Get XY.vi"("VISA In"=w861) -> ("XPosition"=w876:i32, "YPosition"=w875:i32)  [unwired: 2 out]
                    n612 = Build Array (concatenate)(w877, w876, w875) -> (w871:i32[])
                    "TempXYArray" <- w871
                    n613 = local read "TileXYCoordinates"() -> (w872:i32[][])
                    n614 = property on="Tile ROI" class="Bool"() -> ("Disabled"=w868:u8)  [unwired: 2 in, 2 out]
                    n615 = Equal To 0?(x=w868) -> (x = 0?=w867:bool)
                    n616 = Insert Into Array(array=w872, new element=w871) -> (w866:i32[][])  [unwired: 2 in]
                    "TileXYCoordinates" <- w866
                    n617 = Array Size(array=w866) -> (size(s)=w865:i32[])
                    n618 = Index Array(array=w865, index=0) -> (element=w863:i32)
                    n619 = Decrement(x=w863) -> (x-1=w862:i32)
                    n620 = call "subvi Robot Manage ROI Listbox.vi"("ROIListBoxIn"=w870, "ROIName"=w869, "XYListOffset"=w862, "Action"=T17."Add") -> ("ROIListBoxOut"=w878:string[][], "TotalROI"=w874:u32)  [unwired: 5 in]
                    "TotROI" <- w874
                    n621 = Decrement(x=w874) -> (x-1=w873:u32)
                    n622 = property on="ROI List" class="MCListbox (strict)"("Item Names"=w878, "Value"=w873) -> ()  [unwired: 2 in, 2 out]
                    n623 = case shown="False" w867 {
                      frame False {
                        n624 = property on="Tile ROI" class="Bool"("Disabled"=u8 0) -> ()  [unwired: 2 in, 2 out]
                      }
                      frame True {
                      }
                    }
                  }
                }
              }
            }
          }
          frame #3 {
            n625 = case shown="True" "Delete ROI" {
              tunnel: w882 -> [_ w890]
              tunnel: w881 -> [_ w887]
              frame False {
              }
              frame True {
                # "If No ROI, clear offsets"
                # "Highlight the one above deleted ROI"
                n626 = Decrement(x=w887) -> (x-1=w886:i32)
                n627 = call "subvi Robot Manage ROI Listbox.vi"("ROIListBoxIn"=w890, "Selection"=w887, "Action"=T17."Delete") -> ("ROIListBoxOut"=w888:string[][], "TotalROI"=w885:u32)  [unwired: 6 in]
                n628 = local write "TotROI"(w885) -> ()
                n629 = property on="ROI List" class="MCListbox (strict)"("Item Names"=w888, "Value"=w886) -> ()  [unwired: 2 in, 2 out]
                n630 = Equal To 0?(x=w885) -> (x = 0?=w884:bool)
                n631 = case shown="True" w884 {
                  frame False {
                  }
                  frame True {
                    w892 = 0
                    n632 = global write "ProSCI Global.vi" "gGlobalOffsetY"(w892) -> ()
                    n633 = global write "ProSCI Global.vi" "gGlobalOffsetX"(w892) -> ()
                    n634 = local write "OffsetPresent"(FALSE) -> ()
                  }
                }
              }
            }
          }
          frame #4 {
            n635 = case shown="True" "Rename ROI" {
              tunnel: w895 -> [_ w901]
              tunnel: w893 -> [_ w898]
              tunnel: w894 -> [_ w900]
              frame False {
              }
              frame True {
                # "ROI Name\nNot Blank"
                n636 = String Length(string=w898) -> (length=w899:i32)
                n637 = Not Equal To 0?(x=w899) -> (x != 0?=w897:bool)
                n638 = case shown="True" w897 {
                  tunnel: w901 -> [_ w906]
                  tunnel: w898 -> [_ w905]
                  tunnel: w900 -> [_ w904]
                  frame False {
                    n639 = call "Subvi Event Log.vi"("EventNum"=u32 5) -> ()  [unwired: 1 in]
                  }
                  frame True {
                    n640 = call "subvi Robot Manage ROI Listbox.vi"("ROIListBoxIn"=w906, "ROIName"=w905, "Selection"=w904, "Action"=T17."Rename") -> ("ROIListBoxOut"=w903:string[][])  [unwired: 5 in, 1 out]
                    n641 = property on="ROI List" class="MCListbox (strict)"("Item Names"=w903) -> ()  [unwired: 2 in, 2 out]
                  }
                }
              }
            }
          }
          frame #5 {
            n642 = case shown="True" "Tile ROI" {
              tunnel: w909 -> [_ w919]
              tunnel: w908 -> [_ w918]
              frame False {
              }
              frame True {
                n643 = call "subvi Robot Extract ROI Info.vi"("ROIListBoxIn"=w919, "Selection"=w918) -> ("TotalTiles"=w917:u32)  [unwired: 3 out]
                n644 = Greater?(x=w917, y=u32 1) -> (0:w915:bool)
                n645 = case shown="True" w915 {
                  tunnel: [TRUE w925] -> w912
                  tunnel: [2 w924] -> w913
                  tunnel: [0 w923] -> w911
                  frame False {
                  }
                  frame True {
                    n646 = Two Button Dialog(message="Tile Definition Exists for this ROI.\nDo you want to setup tiles again?", 2:"Yes" ("T button name (\"OK\")")) -> (T button?=w926:bool)  [unwired: 1 out]
                    n647 = case shown="True" w926 {
                      tunnel: [FALSE TRUE] -> w925
                      tunnel: [w929 2] -> w924
                      tunnel: [w929 0] -> w923
                      frame False {
                        w929 = 0
                      }
                      frame True {
                      }
                    }
                  }
                }
                n648 = property on="TopEdge" class="Bool"("Visible"=w912, "Blinking"=w912, "Disabled"=w911) -> ()  [unwired: 2 in, 2 out]
                n649 = property on="BotEdge" class="Bool"("Visible"=w912, "Blinking"=w912, "Disabled"=w911) -> ()  [unwired: 2 in, 2 out]
                n650 = property on="LeftEdge" class="Bool"("Visible"=w912, "Blinking"=w912, "Disabled"=w911) -> ()  [unwired: 2 in, 2 out]
                n651 = property on="RightEdge" class="Bool"("Visible"=w912, "Blinking"=w912, "Disabled"=w911) -> ()  [unwired: 2 in, 2 out]
                n652 = property on="Tile ROI" class="Bool"("Disabled"=w913) -> ()  [unwired: 2 in, 2 out]
                "EdgeMarker" <- 0
              }
            }
          }
          frame #6 {
            n653 = case shown="True" "TopEdge" {
              tunnel: w935 -> [_ w951]
              tunnel: w934 -> [_ w949]
              frame False {
              }
              frame True {
                n654 = call "newsubvi Robot Get XY.vi"("VISA In"=w949) -> ("YPosition"=→"TopEdgePos":i32)  [unwired: 3 out]
                n655 = Increment(x=w951) -> (x+1=w950:u8)
                n656 = local write "EdgeMarker"(w950) -> ()
                n657 = property on="TopEdge" class="Bool"("Disabled"=2, "Blinking"=FALSE ("IO Cut Comp")) -> ()  [unwired: 2 in, 2 out]
              }
            }
            n658 = case shown="True" "BotEdge" {
              tunnel: w935 -> [_ w943]
              tunnel: w934 -> [_ w939]
              frame False {
              }
              frame True {
                n659 = call "newsubvi Robot Get XY.vi"("VISA In"=w939) -> ("VISA Out"=w938:refnum<visa-resource-name>, "YPosition"=w940:i32)  [unwired: 2 out]
                n660 = call "newSubvi Safety Check.vi"("VISA In"=w938, "SafetyCheck"=T18."YMax", "YTarget"=w940) -> ("Safe"=w942:bool)  [unwired: 2 in, 2 out]
                n661 = case shown="True" w942 {
                  tunnel: w940 -> [_ w948]
                  tunnel: w943 -> [_ w945]
                  frame False {
                  }
                  frame True {
                    n662 = Increment(x=w945) -> (x+1=w944:u8)
                    n663 = local write "EdgeMarker"(w944) -> ()
                    n664 = property on="BotEdge" class="Bool"("Disabled"=2, "Blinking"=FALSE ("IO Cut Comp")) -> ()  [unwired: 2 in, 2 out]
                    "BotEdgePos" <- w948
                  }
                }
              }
            }
          }
          frame #7 {
            n665 = case shown="True" "LeftEdge" {
              tunnel: w956 -> [_ w970]
              tunnel: w955 -> [_ w966]
              frame False {
              }
              frame True {
                n666 = call "newsubvi Robot Get XY.vi"("VISA In"=w966) -> ("VISA Out"=w965:refnum<visa-resource-name>, "XPosition"=w968:i32)  [unwired: 2 out]
                n667 = call "newSubvi Safety Check.vi"("VISA In"=w965, "SafetyCheck"=T18."XMin", "XTarget"=w968) -> ("Safe"=w967:bool)  [unwired: 2 in, 2 out]
                n668 = case shown="True" w967 {
                  tunnel: w970 -> [_ w973]
                  tunnel: w968 -> [_ w971]
                  frame False {
                  }
                  frame True {
                    n669 = Increment(x=w973) -> (x+1=w972:u8)
                    n670 = local write "EdgeMarker"(w972) -> ()
                    n671 = property on="LeftEdge" class="Bool"("Disabled"=2, "Blinking"=FALSE ("IO Cut Comp")) -> ()  [unwired: 2 in, 2 out]
                    "LtEdgePos" <- w971
                  }
                }
              }
            }
            n672 = case shown="True" "RightEdge" {
              tunnel: w956 -> [_ w961]
              tunnel: w955 -> [_ w959]
              frame False {
              }
              frame True {
                n673 = call "newsubvi Robot Get XY.vi"("VISA In"=w959) -> ("XPosition"=→"RtEdgePos":i32)  [unwired: 3 out]
                n674 = Increment(x=w961) -> (x+1=w960:u8)
                n675 = local write "EdgeMarker"(w960) -> ()
                n676 = property on="RightEdge" class="Bool"("Disabled"=2, "Blinking"=FALSE ("IO Cut Comp")) -> ()  [unwired: 2 in, 2 out]
              }
            }
          }
          frame #8 {
            n677 = Greater Or Equal?(x=w981, y=u8 4) -> (x >= y?=w980:bool)
            n678 = case shown="True" w980 {
              tunnel: w979 -> [_ w995]
              tunnel: w978 -> [_ w994]
              tunnel: w977 -> [_ w993]
              tunnel: w976 -> [_ w992]
              frame False {
              }
              frame True {
                # "Check edges r valid;\nRt>Lt & Bot>Top"
                n679 = local read "TopEdgePos"() -> (w999:i32)
                n680 = local read "BotEdgePos"() -> (w998:i32)
                n681 = local read "RtEdgePos"() -> (w996:i32)
                n682 = local read "LtEdgePos"() -> (w997:i32)
                n683 = Greater Or Equal?(x=w996, y=w997) -> (x >= y?=w991:bool)
                n684 = Greater Or Equal?(x=w998, y=w999) -> (x >= y?=w990:bool)
                n685 = And(x=w991, y=w990) -> (x .and. y?=w1000:bool)
                n686 = case shown="True" w1000 {
                  tunnel: w999 -> [_ w1031]
                  tunnel: w998 -> [_ w1030]
                  tunnel: w997 -> [_ w1029]
                  tunnel: w996 -> [_ w1028]
                  tunnel: w995 -> [_ w1027]
                  tunnel: w994 -> [_ w1026]
                  tunnel: w993 -> [_ w1025]
                  tunnel: w992 -> [_ w1024]
                  tunnel: w991 -> [w1006 _]
                  tunnel: w990 -> [w1005 _]
                  tunnel: [w1010 w1023] -> w989
                  tunnel: [0 w1022] -> w988
                  tunnel: [w1009 w1021] -> w987
                  tunnel: [0 w1020] -> w986
                  tunnel: [w1001 w1019] -> w985
                  tunnel: "MinOverlap" -> [_ w1018]
                  tunnel: "EProfile" -> [_ w1017]
                  frame False {
                    # "Edges Invalid, reset markers"
                    n687 = case shown="False" w1006 {
                      tunnel: [TRUE ("IO Cut Comp") FALSE ("IO Cut Comp")] -> w1010
                      frame False {
                        n688 = call "Subvi Event Log.vi"("EventNum"=u32 6) -> ()  [unwired: 1 in]
                      }
                      frame True {
                      }
                    }
                    n689 = case shown="False" w1005 {
                      tunnel: [TRUE ("IO Cut Comp") FALSE ("IO Cut Comp")] -> w1009
                      frame False {
                        n690 = call "Subvi Event Log.vi"("EventNum"=u32 7) -> ()  [unwired: 1 in]
                      }
                      frame True {
                      }
                    }
                    n691 = Or(x=w1006, y=w1005) -> (x .or. y?=w1004:bool)
                    n692 = Select(t=u8 2 ("EdgeMarker"), s=w1004, f=u8 0 ("EdgeMarker")) -> (s? t:f=w1001:u8)
                  }
                  frame True {
                    n693 = stacked-sequence {
                      seq-local: [w1032 _ _ _] -> [_ w1041 _ _]
                      tunnel: w1031 -> [_ w1056 _ _]
                      tunnel: w1030 -> [_ w1055 _ _]
                      tunnel: w1029 -> [_ w1054 _ _]
                      tunnel: w1028 -> [_ w1053 _ _]
                      tunnel: w1027 -> [_ w1052 _ _]
                      tunnel: w1026 -> [_ w1051 _ _]
                      tunnel: w1025 -> [_ w1046 _ _]
                      tunnel: w1024 -> [_ w1044 _ _]
                      tunnel: [_ _ w1061 _] -> w1023
                      tunnel: [_ _ w1060 _] -> w1022
                      tunnel: [_ _ w1061 _] -> w1021
                      tunnel: [_ _ w1060 _] -> w1020
                      tunnel: [_ _ w1060 _] -> w1019
                      tunnel: w1018 -> [_ w1039 _ _]
                      tunnel: w1017 -> [_ w1038 _ _]
                      frame #0 {
                        n694 = local read "TileXYCoordinates"() -> (w1033:i32[][])
                        n695 = Array Size(array=w1033) -> (size(s)=w1034:i32[])
                        n696 = Index Array(array=w1034, index=0) -> (element=w1032:i32)
                      }
                      frame #1 {
                        n697 = Divide(x="Overlap", y=100.0) -> (x/y=w1058:dbl)
                        n698 = call "subvi Robot Calculate Tile XY.vi"("EProfileMove"=w1038, "OverlapPriority"=w1039, "MinOverlap"=w1058, "Magnification"=w1051, "Objective"=w1052, "Right"=w1053, "Left"=w1054, "Bottom"=w1055, "Top"=w1056) -> ("TileInfo Cluster"=w1050:T20)
                        n699 = local read "TileXYCoordinates"() -> (w1047:i32[][])
                        n700 = Unbundle(w1050) -> ("TileCoordinates"=w1048:i32[][], "XTiles"=w1043:u16, "YTiles"=w1042:u16, "XOverlap"=w1037:dbl, "YOverlap"=w1036:dbl)  [unwired: 1 out]
                        n701 = call "subvi Robot Manage ROI Listbox.vi"("OverlapY"=w1036, "ROIListBoxIn"=w1046, "XYListOffset"=w1041, "TileY"=w1042, "TileX"=w1043, "OverlapX"=w1037, "Selection"=w1044, "Action"=T17."Update Tiles") -> ("ROIListBoxOut"=w1040:string[][])  [unwired: 1 in, 1 out]
                        n702 = property on="ROI List" class="MCListbox (strict)"("Item Names"=w1040) -> ()  [unwired: 2 in, 2 out]
                        n703 = Insert Into Array(array=w1047, new element=w1048) -> (w1049:i32[][])  [unwired: 2 in]
                        n704 = local write "TileXYCoordinates"(w1049) -> ()
                      }
                      frame #2 {
                        w1060 = 0
                        w1061 = FALSE ("IO Cut Comp")
                        # "Make Edge Markers Invisible\nTile ROI Button Enabled\nEdge Marker counter reset to 0"
                        n705 = property on="Tile ROI" class="Bool"("Disabled"=w1060) -> ()  [unwired: 2 in, 2 out]
                      }
                      frame #3 {
                      }
                    }
                  }
                }
                n706 = local write "EdgeMarker"(w985) -> ()
                n707 = property on="RightEdge" class="Bool"("Visible"=w989, "Blinking"=w989, "Disabled"=w988) -> ()  [unwired: 2 in, 2 out]
                n708 = property on="TopEdge" class="Bool"("Visible"=w987, "Blinking"=w987, "Disabled"=w986) -> ()  [unwired: 2 in, 2 out]
                n709 = property on="LeftEdge" class="Bool"("Visible"=w989, "Blinking"=w989, "Disabled"=w988) -> ()  [unwired: 2 in, 2 out]
                n710 = property on="BotEdge" class="Bool"("Visible"=w987, "Blinking"=w987, "Disabled"=w986) -> ()  [unwired: 2 in, 2 out]
              }
            }
          }
          frame #9 {
            # "Pixel Size"
            n711 = global read "ProSCI ConfigGlobal.vi" "gCfgPixelSize"() -> (w1065:dbl[][])
            n712 = Index Array(array=w1065, index (row)=w1063) -> (element=w1066:dbl[])  [unwired: 1 in]
            n713 = Index Array(array=w1066, index=w1064) -> (element=→"Pixel Size":dbl)
          }
        }
      }
    }
    n714 = property on="AbortSeq" class="Bool"("Disabled"=w658) -> ()  [unwired: 2 in, 2 out]
    n715 = case shown="\"Forward\"" w652 {
      frame "Emergency Off", Default {
        n716 = local write "GoingHome"(FALSE) -> ()
        n717 = property on="PauseReset" class="Bool"("Boolean Text.Text"="PAUSE" ("Caption.Text")) -> ()  [unwired: 2 in, 2 out]
      }
      frame "Pause" {
        # "Going Home status unchanged"
      }
      frame "Go Home" {
        n718 = property on="PauseReset" class="Bool"("Boolean Text.Text"="PAUSE" ("Caption.Text")) -> ()  [unwired: 2 in, 2 out]
      }
      frame "Forward" {
      }
    }
    n719 = And(x=w639, y=w648) -> (x .and. y?=w645:bool)
    n720 = Select(t=0, s=w639, f=2) -> (s? t:f=w653:i32)
    n721 = Set Menu Item Info(7:"Load_Protocol" ("item tag"), 9:w639, 10:"Load Protocol" ("item name"), 11:w638) -> ()  [unwired: 1 in, 4 out]
    n722 = case shown="False" w669 {
      tunnel: [w1086 T5."Emergency Off"] -> w667
      tunnel: w668 -> [w1085 _]
      tunnel: "PauseReset" -> [w1084 _]
      tunnel: "Home" -> [w1083 _]
      tunnel: w634 -> [w1082 _]
      tunnel: w675 -> [w1081 w1419]
      tunnel: [w1080 w1419] -> w642
      tunnel: [w1079 w1417] -> w674
      tunnel: w673 -> [w1078 _]
      tunnel: w662 -> [w1077 _]
      tunnel: w662 -> [w1076 _]
      tunnel: [w1075 w1417] -> w671
      tunnel: w672 -> [w1074 _]
      tunnel: w657 -> [w1073 _]
      tunnel: [w1072 w1417] -> w661
      tunnel: w663 -> [w1071 _]
      tunnel: w662 -> [w1070 _]
      tunnel: [w1069 w1416] -> w641
      tunnel: w640 -> [w1068 w1416]
      frame False {
        n723 = local read "IO Comp Mode?"() -> (w1067:bool)
        n724 = case shown="True" w1067 {
          tunnel: [T5."Idle" w1111] -> w1086
          tunnel: w1085 -> [_ w1110]
          tunnel: w1084 -> [_ w1109]
          tunnel: w1083 -> [_ w1108]
          tunnel: w1082 -> [_ w1107]
          tunnel: w1081 -> [w1090 w1106]
          tunnel: [w1090 w1105] -> w1080
          tunnel: [w1088 w1104] -> w1079
          tunnel: w1078 -> [_ w1103]
          tunnel: w1077 -> [_ w1102]
          tunnel: w1076 -> [_ w1101]
          tunnel: [w1088 w1100] -> w1075
          tunnel: w1074 -> [_ w1099]
          tunnel: w1073 -> [_ w1098]
          tunnel: [w1088 w1097] -> w1072
          tunnel: w1071 -> [_ w1096]
          tunnel: w1070 -> [_ w1095]
          tunnel: [w1087 w1094] -> w1069
          tunnel: w1068 -> [w1087 w1093]
          frame False {
            w1088 = 0
          }
          frame True {
            n725 = global read "ProSCI Global.vi" "gNotify"() -> (w1092:enum16{"None", "Email", "SMS", "Both"})
            n726 = Not Equal To 0?(x=w1092) -> (x != 0?=w1091:bool)
            n727 = case shown="\"Forward\"" w1110 {
              tunnel: [T5."Idle" T5."Idle" w1121 w1157 w1179 w1215 w1241 w1264 w1276 w1286 w1294 w1307 w1376 w1382 w1389] -> w1111
              tunnel: w1110 -> [_ _ w1120 w1157 w1178 w1214 w1240 w1264 _ w1285 w1294 _ w1376 w1381 w1395]
              tunnel: w1109 -> [_ _ _ _ w1177 w1216 w1229 _ _ _ _ _ _ _ _]
              tunnel: w1108 -> [_ _ _ _ w1176 w1213 _ _ _ _ _ _ _ _ _]
              tunnel: w1107 -> [_ _ _ _ w1164 _ w1242 _ _ _ _ _ _ _ _]
              tunnel: w1106 -> [_ _ _ _ w1175 w1212 w1239 w1263 w1274 w1284 w1293 w1306 w1375 w1380 w1402]
              tunnel: [0 0 0 0 w1175 w1212 w1239 w1263 w1274 w1284 w1293 w1296 w1375 w1380 w1402] -> w1105
              tunnel: [w1113 w1117 w1129 w1155 w1174 w1211 w1238 w1262 w1275 0 w1292 w1298 w1374 w1379 w1394] -> w1104
              tunnel: w1103 -> [_ _ w1129 w1155 w1174 w1211 w1238 w1262 w1275 _ w1292 w1298 w1374 w1379 w1398]
              tunnel: w1102 -> [_ _ _ _ _ _ _ _ _ _ _ _ _ _ w1397]
              tunnel: w1101 -> [_ _ _ _ w1170 _ _ _ _ _ _ _ _ _ _]
              tunnel: [w1113 w1117 w1128 w1154 w1168 w1210 0 w1261 w1267 w1282 w1291 w1299 w1373 w1378 w1393] -> w1100
              tunnel: w1099 -> [_ _ w1128 w1154 w1167 _ _ w1261 _ w1282 w1291 w1299 w1373 _ w1393]
              tunnel: w1098 -> [_ _ _ _ w1162 _ _ _ _ _ _ w1302 _ _ _]
              tunnel: [w1113 w1117 0 w1153 0 w1210 w1232 w1260 w1267 0 w1290 0 w1372 w1378 0] -> w1097
              tunnel: w1096 -> [_ _ _ w1153 _ _ w1231 w1260 _ _ w1290 _ w1372 _ _]
              tunnel: w1095 -> [_ _ _ _ _ _ w1233 _ _ _ _ _ _ _ _]
              tunnel: [w1112 w1116 w1125 w1152 w1160 w1208 w1228 w1259 w1266 w1279 w1289 w1300 w1371 w1377 w1388] -> w1094
              tunnel: w1093 -> [w1112 w1116 w1125 w1152 w1160 w1208 w1228 w1259 w1265 w1279 w1289 w1300 w1371 w1377 w1388]
              tunnel: w1091 -> [_ _ _ _ w1159 _ w1227 _ _ _ _ w1295 _ _ _]
              frame "Emergency Off", Default {
                w1113 = 0
              }
              frame "Manual" {
                w1117 = 0
              }
              frame "Idle" {
                n728 = Or(x="Sequence", y="Single") -> (x .or. y?=w1123:bool)
                n729 = case shown="True" w1123 {
                  tunnel: "Sequence" -> [_ w1137]
                  tunnel: [w1131 w1133] -> w1121
                  tunnel: w1120 -> [w1131 w1132]
                  frame False {
                  }
                  frame True {
                    n730 = local read "Image"() -> (w1138:bool)
                    n731 = case shown="False" w1138 {
                      tunnel: [TRUE w1143] -> w1136
                      tunnel: [T5."Forward" w1142] -> w1133
                      tunnel: w1132 -> [_ w1141]
                      frame False {
                      }
                      frame True {
                        n732 = call "newSubvi Safety Check.vi"("SafetyCheck"=T14."Exposure") -> ("Safe"=w1144:bool)  [unwired: 4 in, 2 out]
                        n733 = case shown="True" w1144 {
                          tunnel: [FALSE w1149] -> w1143
                          tunnel: [w1146 T5."Forward"] -> w1142
                          tunnel: w1141 -> [w1146 _]
                          frame False {
                          }
                          frame True {
                            w1149 = TRUE
                            n734 = call "Subvi Calculate Exposure Type.vi"("CutsCompleted"=u32 0) -> ("ThisPass"=w1151:u16)
                            n735 = call "Subvi Setup Lamp And Exposure.vi"("PassImageType"=w1151) -> ()
                            "SaveMetadata" <- w1149
                          }
                        }
                      }
                    }
                    n736 = Select(t=w1136, s=w1137, f=FALSE) -> (s? t:f=w1134:bool)
                    "Sequence Cut" <- w1134
                    n737 = global write "ProSCI Global.vi" "gCutSequenceOn"(w1134) -> ()
                  }
                }
                n738 = local write "Imaging Done"(FALSE) -> ()
              }
              frame "Spare 1" {
              }
              frame "Forward" {
                # "Wait before polling cut comp signal. Shouldn't come immediately"
                n739 = Increment(x=w1167) -> (x+1=w1168:i32)
                n740 = Multiply(x="Time Out (sec)", y=1000.0) -> (x*y=w1172:dbl)
                n741 = Multiply(x=w1168, y=w1170) -> (x*y=w1166:u32)
                n742 = global read "ProSCI Global.vi" "gForwardDelay"() -> (w1158:i32)
                n743 = Greater?(x=w1166, y=w1172) -> (0:w1169:bool)
                n744 = Greater?(x=w1166, y=w1158) -> (0:w1163:bool)
                n745 = And(x=w1164, y=w1163) -> (x .and. y?=w1165:bool)
                n746 = case shown="False" w1177 {
                  tunnel: [w1188 T5."Pause"] -> w1179
                  tunnel: w1169 -> [w1187 _]
                  tunnel: w1178 -> [w1186 _]
                  tunnel: w1176 -> [w1181 _]
                  tunnel: w1165 -> [w1185 _]
                  tunnel: w1162 -> [w1183 _]
                  tunnel: w1159 -> [w1180 _]
                  frame False {
                    n747 = Not(x=w1183) -> (.not. x?=w1182:bool)
                    n748 = And(x=w1181, y=w1182) -> (x .and. y?=w1184:bool)
                    n749 = case shown="False" w1184 {
                      tunnel: [w1193 T5."Go Home"] -> w1188
                      tunnel: w1187 -> [w1192 _]
                      tunnel: w1186 -> [w1191 _]
                      tunnel: w1185 -> [w1190 _]
                      tunnel: w1180 -> [w1189 _]
                      frame False {
                        n750 = case shown="True" w1190 {
                          tunnel: [w1196 w1204] -> w1193
                          tunnel: w1192 -> [w1197 _]
                          tunnel: w1191 -> [w1195 _]
                          tunnel: w1189 -> [w1194 _]
                          frame False {
                            n751 = case shown="True" w1197 {
                              tunnel: [w1198 T5."Time Out"] -> w1196
                              tunnel: w1195 -> [w1198 _]
                              tunnel: w1194 -> [_ w1200]
                              frame False {
                              }
                              frame True {
                                n752 = case shown="False" w1200 {
                                frame False {
                                }
                                frame True {
                                n753 = local write "NotifyAbout"(T2."Sec TO" ("NotifyAbout")) -> ()
                                }
                                }
                                n754 = global write "ProSCI Global.vi" "gBrLampOn"(FALSE) -> ()
                                n755 = call "Subvi Event Log.vi"("EventNum"=u32 25) -> ()  [unwired: 1 in]
                              }
                            }
                          }
                          frame True {
                            n756 = flat-sequence {
                              tunnel: [T5."Cut Complete"] -> w1204
                              frame #0 {
                              }
                              frame #1 {
                              }
                            }
                          }
                        }
                      }
                      frame True {
                      }
                    }
                  }
                  frame True {
                  }
                }
              }
              frame "Pause" {
                w1210 = 0
                n757 = case shown="True" w1216 {
                  tunnel: [w1219 w1223] -> w1215
                  tunnel: w1214 -> [w1218 _]
                  tunnel: w1213 -> [w1217 _]
                  frame False {
                    n758 = case shown="False" w1217 {
                      tunnel: [w1221 T5."Go Home"] -> w1219
                      tunnel: w1218 -> [w1221 _]
                      frame False {
                      }
                      frame True {
                      }
                    }
                    n759 = property on="PauseReset" class="Bool"("Boolean Text.Text"="RESUME" ("Caption.Text")) -> ()  [unwired: 2 in, 2 out]
                  }
                  frame True {
                    n760 = local read "GoingHome"() -> (w1224:bool)
                    n761 = Select(t=T5."Go Home", s=w1224, f=T5."Forward") -> (s? t:f=w1223:T5)
                  }
                }
                n762 = global write "ProSCI Global.vi" "gCutSequenceOn"(FALSE) -> ()
              }
              frame "Go Home" {
                # "Check for\nTimeout"
                n763 = Increment(x=w1231) -> (x+1=w1232:i32)
                n764 = Multiply(x=w1232, y=w1233) -> (x*y=w1235:u32)
                n765 = Greater?(x=w1235, y=u32 8000) -> (0:w1230:bool)
                n766 = case shown="True" w1242 {
                  tunnel: [w1246 T5."Idle"] -> w1241
                  tunnel: w1240 -> [w1245 _]
                  tunnel: w1230 -> [w1247 _]
                  tunnel: w1229 -> [w1244 _]
                  tunnel: w1227 -> [w1243 _]
                  frame False {
                    n767 = case shown="False" w1244 {
                      tunnel: w1247 -> [w1251 _]
                      tunnel: [w1250 T5."Pause"] -> w1246
                      tunnel: w1245 -> [w1249 _]
                      tunnel: w1243 -> [w1248 _]
                      frame False {
                        n768 = case shown="True" w1251 {
                          tunnel: [w1252 T5."Time Out"] -> w1250
                          tunnel: w1249 -> [w1252 _]
                          tunnel: w1248 -> [_ w1253]
                          frame False {
                          }
                          frame True {
                            n769 = case shown="True" w1253 {
                              frame False {
                              }
                              frame True {
                                n770 = local write "NotifyAbout"(T2."Sec TO" ("NotifyAbout")) -> ()
                              }
                            }
                            n771 = call "Subvi Event Log.vi"("EventNum"=u32 24) -> ()  [unwired: 1 in]
                          }
                        }
                      }
                      frame True {
                      }
                    }
                  }
                  frame True {
                  }
                }
                "GoingHome" <- TRUE
              }
              frame "Spare 2" {
              }
              frame "Cut Complete" {
                w1267 = 0
                n772 = Increment(x="ImageSkipNum") -> (x+1=w1268:i32)
                n773 = Increment(x=w1265) -> (x+1=w1266:i32)
                n774 = Quotient & Remainder(x=w1274, y=w1268) -> (x-y*floor(x/y)=w1271:i32)  [unwired: 1 out]
                n775 = Equal To 0?(x=w1271) -> (x = 0?=w1270:bool)
                n776 = And(x="Image", y=w1270) -> (x .and. y?=w1272:bool)
                n777 = case shown="True" w1272 {
                  tunnel: [T5."Calculate Cuts" T5."Delay Before Imaging"] -> w1276
                  frame False {
                  }
                  frame True {
                  }
                }
              }
              frame "Imaging" {
                n778 = local read "Imaging Done"() -> (w1281:bool)
                n779 = case shown="True" w1281 {
                  tunnel: [w1287 T5."Calculate Cuts"] -> w1286
                  tunnel: w1285 -> [w1287 _]
                  frame False {
                  }
                  frame True {
                  }
                }
              }
              frame "Spare 3" {
              }
              frame "Calculate Cuts" {
                n780 = Not(x=w1302) -> (.not. x?=w1308:bool)
                n781 = Increment(x=w1306) -> (x+1=w1296:i32)
                "CutsCompletedLast" <- w1296
                n782 = Greater Or Equal?(x=w1296, y="Total Cuts") -> (x >= y?=w1309:bool)
                n783 = Or(x=w1308, y=w1309) -> (x .or. y?=w1305:bool)
                n784 = Or(x="AbortSeq", y=w1305) -> (x .or. y?=w1304:bool)
                n785 = case shown="False" w1304 {
                  tunnel: [T5."Forward" T5."Idle"] -> w1307
                  tunnel: w1296 -> [w1312 w1358]
                  tunnel: w1295 -> [w1311 w1357]
                  tunnel: "AbortSeq" -> [_ w1356]
                  frame False {
                    n786 = stacked-sequence {
                      tunnel: w1312 -> [w1315 w1347]
                      tunnel: w1311 -> [w1314 _]
                      tunnel: w1311 -> [_ w1348]
                      frame #0 {
                        n787 = local read "Image"() -> (w1316:bool)
                        n788 = case shown="False" w1316 {
                          tunnel: w1315 -> [_ w1318]
                          tunnel: w1314 -> [_ w1317]
                          frame False {
                          }
                          frame True {
                            n789 = stacked-sequence {
                              tunnel: w1318 -> [w1319 w1320 _]
                              tunnel: w1317 -> [_ _ _]
                              frame #0 {
                                # "Imaging Mode for this & next\npass"
                                n790 = call "Subvi Calculate Exposure Type.vi"("CutsCompleted"=w1319) -> ()  [unwired: 1 out]
                              }
                              frame #1 {
                                n791 = case shown="False" "Auto Offset" {
                                tunnel: w1320 -> [_ w1322]
                                frame False {
                                }
                                frame True {
                                n792 = stacked-sequence {
                                seq-local: [w1323 _] -> [_ w1328]
                                tunnel: w1322 -> [w1326 w1327]
                                frame #0 {
                                # "Add Autocalculated\nOffset if this is the section to apply it."
                                n793 = local read "OffsetSlice"() -> (w1325:u32)
                                n794 = Quotient & Remainder(x=w1326, y=w1325) -> (x-y*floor(x/y)=w1324:u32)  [unwired: 1 out]
                                n795 = Equal To 0?(x=w1324) -> (x = 0?=w1323:bool)
                                }
                                frame #1 {
                                n796 = case shown="True" w1328 {
                                tunnel: w1327 -> [_ w1329]
                                frame False {
                                }
                                frame True {
                                n797 = stacked-sequence {
                                seq-local: [w1330 _ _] -> [_ w1337 _]
                                seq-local: [_ w1335 _] -> [_ _ w1339]
                                tunnel: w1329 -> [_ _ _]
                                frame #0 {
                                n798 = local read "TileXYCoordinates"() -> (w1333:i32[][])
                                n799 = local read "AutoXOffset"() -> (w1330:i32)
                                n800 = call "Subvi Add Offset to XY Coordinates.vi"("YOffsetIn"=0, "XOffsetIn"=w1330, "TileXYCoordinatesIn"=w1333) -> ("TileXYCoordinatesOut"=w1332:i32[][])
                                n801 = local write "TileXYCoordinates"(w1332) -> ()
                                }
                                frame #1 {
                                n802 = local read "SecNumInFile"() -> (w1334:u32)
                                n803 = Increment(x=w1334) -> (x+1=w1335:u32)
                                n804 = call "Subvi Write Metadata.vi"("YOffsetIn"=0, "XOffsetIn"=w1337, "Next Cut"=w1335, "Store Offset (F)"=TRUE) -> ()  [unwired: 4 in]
                                }
                                frame #2 {
                                n805 = Number To Decimal String(number=w1339) -> (decimal integer string=w1341:string)  [unwired: 1 out]
                                n806 = Concatenate Strings("Auto Offset Applied @ File  ", w1341) -> (w1342:string)
                                n807 = call "Subvi Event Log.vi"("CustomMessage"=w1342) -> ()  [unwired: 1 in]
                                }
                                }
                                }
                                }
                                }
                                }
                                }
                                }
                              }
                              frame #2 {
                                # "Setup Robot"
                                n808 = local read "TotROI"() -> (w1344:i32)
                                n809 = Not Equal To 0?(x=w1344) -> (x != 0?=w1343:bool)
                                n810 = case shown="True" w1343 {
                                frame False {
                                }
                                frame True {
                                n811 = stacked-sequence {
                                frame #0 {
                                n812 = property on="ROI List" class="MCListbox (strict)"("Value"=0 ("ROI List")) -> ()  [unwired: 2 in, 2 out]
                                }
                                frame #1 {
                                n813 = local write "MoveTo ROI"(TRUE) -> ()
                                }
                                }
                                }
                                }
                              }
                            }
                          }
                        }
                      }
                      frame #1 {
                        n814 = case shown="False" w1348 {
                          tunnel: w1347 -> [_ w1355]
                          frame False {
                          }
                          frame True {
                            # "Send Notification to User"
                            n815 = global read "ProSCI Global.vi" "gNotifyEvery"() -> (w1354:u32)
                            n816 = Quotient & Remainder(x=w1355, y=w1354) -> (x-y*floor(x/y)=w1353:u32)  [unwired: 1 out]
                            n817 = Equal To 0?(x=w1353) -> (x = 0?=w1352:bool)
                            n818 = Select(t=T19."In Progress" ("NotifyAbout"), s=w1352, f=T19."Nothing" ("NotifyAbout")) -> (s? t:f=→"NotifyAbout":T19)
                          }
                        }
                      }
                    }
                  }
                  frame True {
                    n819 = stacked-sequence {
                      tunnel: w1358 -> [w1362 _ _]
                      tunnel: w1357 -> [_ _ w1366]
                      tunnel: w1356 -> [_ _ w1365]
                      frame #0 {
                        n820 = local read "FileNumStart"() -> (w1361:i32)
                        n821 = Add(x=w1361, y=w1362) -> (x+y=w1360:i32)
                        n822 = local write "FileNumStart"(w1360) -> ()
                      }
                      frame #1 {
                        w1364 = u32 0 ("Present Cuts")
                        w1363 = FALSE
                        n823 = property on="Sequence Cut" class="Bool (strict)"("Value"=w1363) -> ()  [unwired: 2 in, 2 out]
                        n824 = global write "ProSCI Global.vi" "gBrLampOn"(w1363) -> ()
                        n825 = global write "ProSCI Global.vi" "gFlLampOn"(w1363) -> ()
                        n826 = property on="Present Cuts" class="DigNum (strict)"("Value"=w1364) -> ()  [unwired: 2 in, 2 out]
                        n827 = global write "ProSCI Global.vi" "gCutSequenceOn"(w1363) -> ()
                        n828 = local write "SecNumInFile"(w1364) -> ()
                      }
                      frame #2 {
                        n829 = case shown="False" w1366 {
                          tunnel: w1365 -> [_ w1370]
                          frame False {
                          }
                          frame True {
                            # "Send Notification to User"
                            n830 = Select(t=T19."Aborted" ("NotifyAbout"), s=w1370, f=T19."Completed" ("NotifyAbout")) -> (s? t:f=w1367:T19)
                            n831 = local write "NotifyAbout"(w1367) -> ()
                          }
                        }
                      }
                    }
                  }
                }
                n832 = local write "Imaging Done"(FALSE ("Imaging Done")) -> ()
              }
              frame "Spare 4" {
              }
              frame "Time Out" {
                w1378 = 0
                n833 = case shown="True" "Sys Reset" {
                  tunnel: [w1384 T5."Idle"] -> w1382
                  tunnel: w1381 -> [w1384 _]
                  frame False {
                  }
                  frame True {
                  }
                }
              }
              frame "Delay Before Imaging" {
                # "Setup File Number"
                n834 = global read "ProSCI Global.vi" "gPreImagingDelay"() -> (w1386:i32)
                n835 = Increment(x=w1398) -> (x+1=w1394:i32)
                n836 = Multiply(x=w1394, y=w1397) -> (x*y=w1400:u32)
                n837 = Multiply(x="Image Delay (sec)", y=1000.0) -> ()  [unwired: 1 out]
                n838 = local read "Camera Prog. OK"() -> (w1391:bool)
                n839 = Greater?(x=w1400, y=w1386) -> (0:w1390:bool)
                n840 = And(x=w1390, y=w1391) -> (x .and. y?=w1387:bool)
                n841 = case shown="True" w1387 {
                  frame False {
                  }
                  frame True {
                    n842 = local read "Present Cuts"() -> (w1404:u32)
                    n843 = case shown="\"With Section No.\", Default" "FileNumbering" {
                      tunnel: "FileNumStart" -> [w1409 w1415]
                      tunnel: w1404 -> [w1408 w1414]
                      tunnel: [w1407 w1413] -> w1403
                      frame "Continuous" {
                        n844 = local read "ImageSkipNum"() -> (w1410:i32)
                        n845 = Increment(x=w1410) -> (x+1=w1412:i32)
                        n846 = Quotient & Remainder(x=w1408, y=w1412) -> (floor(x/y)=w1411:u32)  [unwired: 1 out]
                        n847 = Add(x=w1409, y=w1411) -> (x+y=w1407:u32)
                      }
                      frame "With Section No.", Default {
                        n848 = Add(x=w1415, y=w1414) -> (x+y=w1413:u32)
                      }
                    }
                    "SecNumInFile" <- w1403
                  }
                }
                n849 = Select(t=T5."Imaging", s=w1387, f=w1395) -> (s? t:f=w1389:T5)
              }
            }
          }
        }
      }
      frame True {
        w1417 = 0
      }
    }
    "Current State" <- w667
    "Present Cuts" <- w642
    "InFwdState" <- w671
    "InDelayState" <- w674
    "InGoHomeState" <- w661
    "TotalSessionCuts" <- w641
    n850 = Wait Until Next ms Multiple(millisecond multiple=w662) -> ()  [unwired: 1 out]
    n851 = Select(t=0, s=w645, f=2) -> (s? t:f=w644:i32)
    n852 = property on="Single" class="Bool"("Disabled"=w653) -> ()  [unwired: 2 in, 2 out]
    n853 = property on="Sequence" class="Bool"("Disabled"=w644) -> ()  [unwired: 2 in, 2 out]
    n854 = case shown="\"Emergency Off\", Default" w652 {
      tunnel: [w679 1 w682 0] -> w651
      tunnel: [w679 0 w682 1] -> w650
      frame "Emergency Off", Default {
        w679 = 1
      }
      frame "Idle" {
      }
      frame "Forward", "Pause" {
        w682 = 0
      }
      frame "Go Home" {
      }
    }
    n855 = case shown="\"Idle\", Default" w652 {
      frame "Idle", Default {
      }
      frame "Emergency Off", "Manual", "Go Home", "Time Out" {
        w685 = FALSE
        n856 = global write "ProSCI Global.vi" "gCutSequenceOn"(w685) -> ()
        n857 = local write "Sequence Cut"(w685) -> ()
      }
    }
    n858 = property on="Home" class="Bool"("Disabled"=w650) -> ()  [unwired: 2 in, 2 out]
    n859 = property on="PauseReset" class="Bool"("Disabled"=w651) -> ()  [unwired: 2 in, 2 out]
    n860 = local read "stop"() -> (w670:bool)
    n861 = Not Equal?(x=w668, y=w667) -> (x != y?=w666:bool)
    n862 = global write "ProSCI Global.vi" "gCutsCompleted"(w642) -> ()
    n863 = And(x=w666, y=TRUE) -> (x .and. y?=w643:bool)
    n864 = case shown="True" w643 {
      frame False {
      }
      frame True {
        "StXition" <- TRUE
      }
    }
  }
  n865 = while {
    tunnel: w6 -> [w1425]
    tunnel: w5 -> [w1424]
    tunnel: w4 -> [w1423]
    tunnel: [w1422] -> w3
    tunnel: [w1421] -> w2
    tunnel: [w1420] -> w1
    stop <- w1428 stop-if-true
    n866 = local read "Start Cut"() -> (w1427:bool)
    n867 = Wait (ms)(milliseconds to wait=u32 5) -> ()  [unwired: 1 out]
    n868 = case shown="True" w1427 {
      tunnel: w1425 -> [w1431 w1437]
      tunnel: w1424 -> [w1430 w1436]
      tunnel: w1423 -> [w1429 w1435]
      tunnel: [w1431 w1434] -> w1422
      tunnel: [w1430 w1433] -> w1421
      tunnel: [w1429 w1432] -> w1420
      frame False {
      }
      frame True {
        n869 = stacked-sequence {
          tunnel: [_ FALSE _] -> _
          tunnel: w1437 -> [_ w1445 _]
          tunnel: w1436 -> [_ w1444 _]
          tunnel: w1435 -> [_ w1443 _]
          tunnel: [_ w1442 _] -> w1434
          tunnel: [_ w1441 _] -> w1433
          tunnel: [_ w1440 _] -> w1432
          frame #0 {
            n870 = local write "Start Cut"(FALSE) -> ()
            n871 = local write "IO Cut Comp"(FALSE ("UseTCP")) -> ()
          }
          frame #1 {
            n872 = call "MoveToTop_ProSCI2.vi"("task out"=w1445, "error out 2"=w1444, "VISA resource name out"=w1443) -> ("task out 2"=w1442:refnum<k21>, "error out"=w1441:errorcluster, "VISA resource name out 2"=w1440:refnum<visa-resource-name>)  [unwired: 3 in]
          }
          frame #2 {
            "IO Cut Comp" <- TRUE ("UseTCP")
          }
        }
      }
    }
    n873 = control-ref of="Start Cut Output"() -> ()  [unwired: 1 out]
    n874 = local read "stop"() -> (w1428:bool)
  }
  n875 = call "cryostat move close.vi"("VISA resource name"=w1, "error in"=w2, "task in"=w3) -> ()  [unwired: 9 in]
  n876 = while {
    stop <- w1450 stop-if-true
    n877 = local read "Stop Cut"() -> (w1449:bool)
    n878 = Wait (ms)(milliseconds to wait=u32 5) -> ()  [unwired: 1 out]
    n879 = control-ref of="Stop Cut Output"() -> (w1451:refnum<vi>)
    n880 = case shown="False" w1449 {
      tunnel: w1449 -> [_ w1453]
      tunnel: w1451 -> [_ w1452]
      frame False {
      }
      frame True {
        n881 = call "Subvi Boolean Stretcher Copy2.vi"("Bool Refnum"=w1452, "Trigger"=w1453, "Delay Cycles"=u32 10) -> ()
      }
    }
    n882 = local read "stop"() -> (w1450:bool)
  }
  n883 = while {
    stop <- w1457 stop-if-true
    n884 = local read "Go Home"() -> (w1456:bool)
    n885 = Wait (ms)(milliseconds to wait=u32 5) -> ()  [unwired: 1 out]
    n886 = control-ref of="Go Home Output"() -> (w1458:refnum<vi>)
    n887 = case shown="False" w1456 {
      tunnel: w1456 -> [_ w1459]
      tunnel: w1458 -> [_ w1460]
      frame False {
      }
      frame True {
        n888 = call "Subvi Boolean Stretcher Copy3.vi"("Bool Refnum"=w1460, "Trigger"=w1459, "Delay Cycles"=u32 10) -> ()
      }
    }
    n889 = local read "stop"() -> (w1457:bool)
  }
  n890 = Tick Count (ms)() -> (millisecond timer value=w13:u32)
  n891 = local read "RobotOnline"() -> (w11:bool)
  n892 = while {
    tunnel: [w1476] -> w14
    shift-right: [w1469] -> _
    shift-left: w13 -> [w1468]
    stop <- w1476 stop-if-true
    # "Dummy Code to force a read"
    # "Slow Loop for Monitoring; every 10 seconds"
    n893 = local read "SaveMetadata"() -> (w1479:bool)
    n894 = local read "UpdateMetadata"() -> (w1477:bool)
    n895 = Or(x="BrConnectButton", y="BrDisonnectButton") -> ()  [unwired: 1 out]
    n896 = Wait (ms)(milliseconds to wait=u32 1000) -> ()  [unwired: 1 out]
    n897 = Tick Count (ms)() -> (millisecond timer value=w1471:u32)
    n898 = Or(x=w1479, y=w1477) -> (x .or. y?=w1478:bool)
    n899 = Subtract(x=w1471, y=w1468) -> (x-y=w1473:u32)
    n900 = Multiply(x=w1473, y=1.0) -> (x*y=w1475:dbl)
    n901 = global read "ProSCI Global.vi" "gNotify"() -> (w1463:enum16{"None", "Email", "SMS", "Both"})
    n902 = case shown="False" "Notify" {
      frame False {
      }
      frame True {
        n903 = call "Subvi Email Settings.vi"() -> ()  [unwired: 1 out]
      }
    }
    n904 = case shown="True" w1478 {
      tunnel: w1477 -> [_ w1500]
      frame False {
      }
      frame True {
        n905 = stacked-sequence {
          tunnel: w1500 -> [w1504 _]
          frame #0 {
            n906 = property on="Magnification" class="CmbBox"() -> ("Strings []"=w1513:string[], "Value"=w1514:string)  [unwired: 2 in, 2 out]
            n907 = property on="Objective" class="CmbBox"() -> ("Strings []"=w1516:string[], "Value"=w1517:string)  [unwired: 2 in, 2 out]
            n908 = Decimal String To Number(string=w1514) -> (number=w1512:i32)  [unwired: 3 out]
            n909 = Decimal String To Number(string=w1517) -> (number=w1515:i32)  [unwired: 3 out]
            n910 = Index Array(array=w1513, index=w1512) -> (element=w1505:string)
            n911 = Index Array(array=w1516, index=w1515) -> (element=w1506:string)
            n912 = Bundle("User"="User", "PI"="PI", "OpSpecimen"="OpSpecimen", "OpSliceThk"="OpSliceThk", "OpNotes"="OpNotes", w1506, w1505) -> (w1502:T21)  [unwired: 1 out]
            n913 = local read "TileXYCoordinates"() -> (w1501:i32[][])
            n914 = property on="ROI List" class="MCListbox (strict)"() -> ("Item Names"=w1503:string[][])  [unwired: 2 in, 2 out]
            n915 = call "Subvi Write Metadata.vi"("TileXYCoordinates"=w1501, "UserFields"=w1502, "ROIListBoxIn"=w1503, "Update (F)"=w1504) -> ()  [unwired: 4 in]
          }
          frame #1 {
            w1518 = FALSE
            n916 = local write "UpdateMetadata"(w1518) -> ()
            n917 = local write "SaveMetadata"(w1518) -> ()
          }
        }
      }
    }
    n918 = Absolute Value(x=w1475) -> (abs(x)=w1472:dbl)
    n919 = Greater?(x=w1472, y=10000.0) -> (0:w1467:bool)
    n920 = Select(t=w1471, s=w1467, f=w1468) -> (s? t:f=w1469:u32)
    n921 = Not Equal To 0?(x=w1463) -> (x != 0?=w1462:bool)
    n922 = Or(x="FlConnectButton", y="FlDisonnectButton") -> ()  [unwired: 1 out]
    n923 = local read "BrConnection"() -> (w1466:bool)
    n924 = And(x=w1466, y=w1467) -> (x .and. y?=w1465:bool)
    n925 = case shown="False" w1462 {
      frame False {
      }
      frame True {
        n926 = local read "NotifyAbout"() -> (w1487:T2)
        n927 = Not Equal?(x=w1487, y=T19."Nothing" ("NotifyAbout")) -> (x != y?=w1488:bool)
        n928 = case shown="False" w1488 {
          tunnel: w1487 -> [_ w1490]
          frame False {
          }
          frame True {
            n929 = stacked-sequence {
              tunnel: w1490 -> [w1494 _]
              frame #0 {
                # "Send Notification"
                n930 = local read "CutsCompletedLast"() -> (w1491:u32)
                n931 = local read "Total Cuts"() -> (w1493:u32)
                n932 = local read "Image"() -> (w1492:bool)
                n933 = call "Subvi Notify User.vi"("Imaging"=w1492, "PresentCutsIn"=w1491, "TotalCutsIn"=w1493, "NotifyAbout"=w1494) -> ("Error"=w1498:bool)
                n934 = Select(t=u32 23 ("EventNum"), s=w1498, f=u32 22 ("EventNum")) -> (s? t:f=w1495:u32)
                n935 = call "Subvi Event Log.vi"("EventNum"=w1495) -> ()  [unwired: 1 in]
              }
              frame #1 {
                # "Reset Notification Flag"
                n936 = local write "NotifyAbout"(T19."Nothing" ("NotifyAbout")) -> ()
              }
            }
          }
        }
      }
    }
    n937 = case shown="True" w1465 {
      frame False {
      }
      frame True {
        n938 = local read "Br VISA Ref"() -> (w1519:refnum<visa-resource-name>)
        n939 = call "subDCRStatus.vi"("VISA resource name"=w1519) -> ("StatusCode"=w1521:u8)  [unwired: 1 out]
        n940 = local write "BrLampStatus"(w1521) -> ()
        n941 = Equal?(x=w1521, y=u8 1) -> (x = y?=w1520:bool)
        n942 = Not(x=w1520) -> (.not. x?=w1522:bool)
        n943 = local write "BrConnection"(w1522) -> ()
      }
    }
    n944 = Get Date/Time String() -> (date string=→"ExpDate":string, time string=→"ExpTime":string)  [unwired: 3 out]
    n945 = global read "ProSCI Global.vi" "gStop All"() -> (w1476:bool)
  }
  n946 = local read "BrConnection"() -> (w17:bool)
  n947 = while {
    stop <- w1524 stop-if-true
    n948 = call "QCameraV1_0.vi"() -> ("stopped"=w1524:bool)
  }
  n949 = And(x=w12, y=w11) -> (x .and. y?=w10:bool)
  n950 = case shown="True" w17 {
    tunnel: w21 -> [_ w1526]
    tunnel: w20 -> [_ w1525]
    frame False {
    }
    frame True {
      # "Note:Closing the serial port allows it to be used by other applications without\nquitting LabVIEW."
      # "Close session to port."
      n951 = VISA Close(VISA resource name=w1526, error in (no error)=w1525) -> (error out=w1527:errorcluster)
      n952 = call <vilib>:"Simple Error Handler.vi"("error in (no error)"=w1527) -> ()  [unwired: 1 in, 8 out]
    }
  }
  n953 = case shown="True" w10 {
    tunnel: w9 -> [_ w1528]
    frame False {
    }
    frame True {
      n954 = VISA Write(VISA resource name=w1528, write buffer="Q") -> (VISA resource name out=w1530:refnum<visa-resource-name>, error out=w1531:errorcluster)  [unwired: 1 in, 1 out]
      n955 = VISA Close(VISA resource name=w1530, error in (no error)=w1531) -> ()  [unwired: 1 out]
    }
  }
  n956 = property class="App"() -> ("Application:Kind"=w15:T22)  [unwired: 2 in, 2 out]
  n957 = case shown="\"Run Time System\"" w15 {
    tunnel: w14 -> [_ w1532]
    frame "invalid app kind", Default {
    }
    frame "Run Time System" {
      n958 = Quit LabVIEW(quit? (T)=w1532) -> ()
    }
  }
